vi "Testing.vi"() -> ()   [LabVIEW 2021]
uses:
  typeDefs/Esophogeal_Software_States.ctl
  <vilib>/Utility/miscctls.llb/LVAllMonitorsDisplayTypeDef.ctl
  <vilib>/DAQmx/read.llb/DAQmx Read (Digital 1D Bool NChan 1Samp 1Line).vi
  <extravilib>/ChannelInstances/Tag-bool/Read With Abort.vi
  <extravilib>/ChannelInstances/High Speed Stream-str/_Read For Replicate.vi
  <extravilib>/ChannelInstances/High Speed Stream-a[.,.](u32)/_Read For Replicate.vi
  <extravilib>/ChannelInstances/Tag-bool/Write With Abort.vi
  <extravilib>/ChannelInstances/High Speed Stream-a[.,.](u8)/_Read For Replicate.vi
  <vilib>/DAQmx/create/channels.llb/DAQmx Create Channel (DI-Digital Input).vi
  <extravilib>/ChannelInstances/Tag-bool/Instantiate.vi
  <extravilib>/ChannelInstances/Tag-bool/EndpointRead.vi
  <extravilib>/ChannelInstances/High Speed Stream-str/Instantiate.vi
  <extravilib>/ChannelInstances/High Speed Stream-a[.,.](u32)/Instantiate.vi
  <extravilib>/ChannelInstances/High Speed Stream-str/)Channel.vi
  <extravilib>/ChannelInstances/High Speed Stream-str/Abort Signal/Init Signal.vi
  <extravilib>/ChannelInstances/High Speed Stream-a[.,.](u32)/)Channel.vi
  <extravilib>/ChannelInstances/High Speed Stream-a[.,.](u32)/Abort Signal/Init Signal.vi
  <vilib>/DAQmx/miscellaneous.llb/DAQmx Fill In Error Info.vi
  <extravilib>/ChannelInstances/Tag-bool/Endpoint.vi
  <extravilib>/ChannelInstances/High Speed Stream-a[.,.](u8)/Instantiate.vi
  <extravilib>/ChannelInstances/High Speed Stream-a[.,.](u8)/)Channel.vi
  <extravilib>/ChannelInstances/High Speed Stream-a[.,.](u8)/Abort Signal/Init Signal.vi
  <vilib>/vision/driver/NI_Vision_Acquisition_Software.lvlib
  <resource>/objmgr/imaqdx.rc
  <extravilib>/ChannelInstances/High Speed Stream-a[.,.](u8).lvlib
  <extravilib>/ChannelInstances/High Speed Stream-str.lvlib
  <vilib>/vision/NI_Vision_Development_Module.lvlib
  <extravilib>/ChannelInstances/High Speed Stream-a[.,.](u32).lvlib
  <extravilib>/ChannelInstances/Tag-bool.lvlib
panel:
  out "Pause Status":bool
  in  "Tab Control":enum32{"Main Page", "Image Session Info"}(tab)
  in  "MTN Threshold:":enum16{"15.9", "24.0"}(ring)
  out "Endoscope Feed":T1(plugin-control)
  in  "Calibrate":bool
  out "Image Analysis Meter":dbl(slide) scale=0.0..100.0
  out "Saved Imaged Number":i32=1 caption="Number of Images Saved"
  out "Image Save Notification":string
  in  "Auto Gain":bool=TRUE
  in  "Auto Exposure":bool=TRUE
  in  "Save Button":bool
  out "Recording":bool
  in  "Play Button":bool
  in  "Pause Button":bool
  in  "Close Program":bool
  in  "HRME Gain":dbl(slide)=18.0 scale=0.0..30.0
  in  "HRME Exposure":dbl(slide)=7000.0 scale=100.0..80000.0
  out "HRME Image":T1(plugin-control)
  out "Software States":T2
  out "HRME Path":path
  out "HRME Scores":path
  out "Representative Images":path
  out "error out":errorcluster
  out "Patient Folder":path
  in  "Command File Location":path=path "C:/Users/EsophaHRME_Dell2/Documents/GitHub/Esophageal_HRME_Software/EsophagealDeployment/Multi_Task_Network/CommandFiles/LabVIEW/cmds.json"
  out "Display:All Monitors":T3
  out "Width":i16
  out "Height":i16=960
  out "WideField Path":path
  in  "Python Module Path":path=path "C:/Users/EsophaHRME_Dell2/Documents/GitHub/Esophageal_HRME_Software/EsophagealDeployment/Multi_Task_Network/mainv6.py"
  out "Log File Out":refnum<file>
  out "Timestamp":string
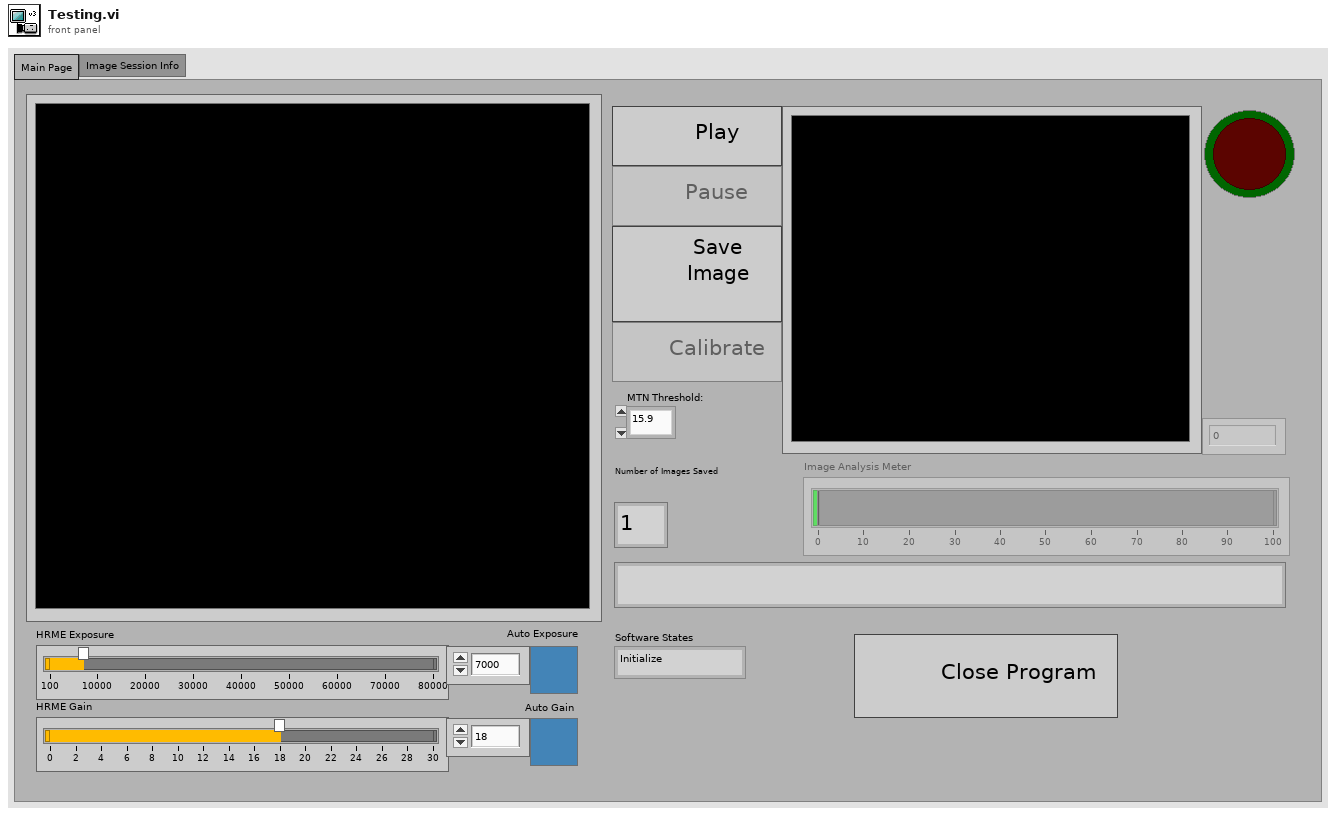
[diagram p1: front panel]
types:
  T1 = typedef "IMAQ Image.ctl" = refnum<image>
  T2 = typedef "Esophogeal_Software_States.ctl" = enum16{"Initialize", "Image Prep Screen", "Imaging", "Image Pause Screen", "Endo Only Saving", "Exit"}
  T3 = typedef "LVAllMonitorsDisplayTypeDef.ctl" = cluster{"Bounds":cluster{"Left":i16, "Top":i16, "Right":i16, "Bottom":i16}, "Depth":i16}[]
  T4 = enum8{"Enabled", "Disabled", "Disabled and Grayed Out"}
  T5 = enum16{"open", "replace", "create", "open or create", "replace or create", "replace or create with confirmation"}
  T6 = cluster{"Source":string, "Destination":string, "CMD":string, "Time":string}
  T7 = cluster{"Left":i32, "Top":i32, "Right":i32, "Bottom":i32}
  T8 = typedef "IMAQdx.ctl" = refnum<k21>
  T9 = cluster{"Bounds":cluster{"Left":i16, "Top":i16, "Right":i16, "Bottom":i16}, "Depth":i16}
  T10 = cluster{"Left":i16, "Top":i16, "Right":i16, "Bottom":i16}
  T11 = typedef "Image Type" = u32
  T12 = typedef "Tag-bool.lvlib/))Channel.ctl" = refnum<queue>
  T13 = typedef "ROI Descriptor" = cluster{"Global Rectangle":i32[], "Contours":cluster{"ID":enum32{"External", "Internal"}, "Type":u32, "Coordinates":i32[]}[]}
  T14 = typedef "High Speed Stream-a[.,.](u32).lvlib/)Channel.ctl" = refnum<queue>
  T15 = typedef "High Speed Stream-str.lvlib/)Channel.ctl" = refnum<queue>
  T16 = typedef "High Speed Stream-a[.,.](u8).lvlib/)Channel.ctl" = refnum<queue>
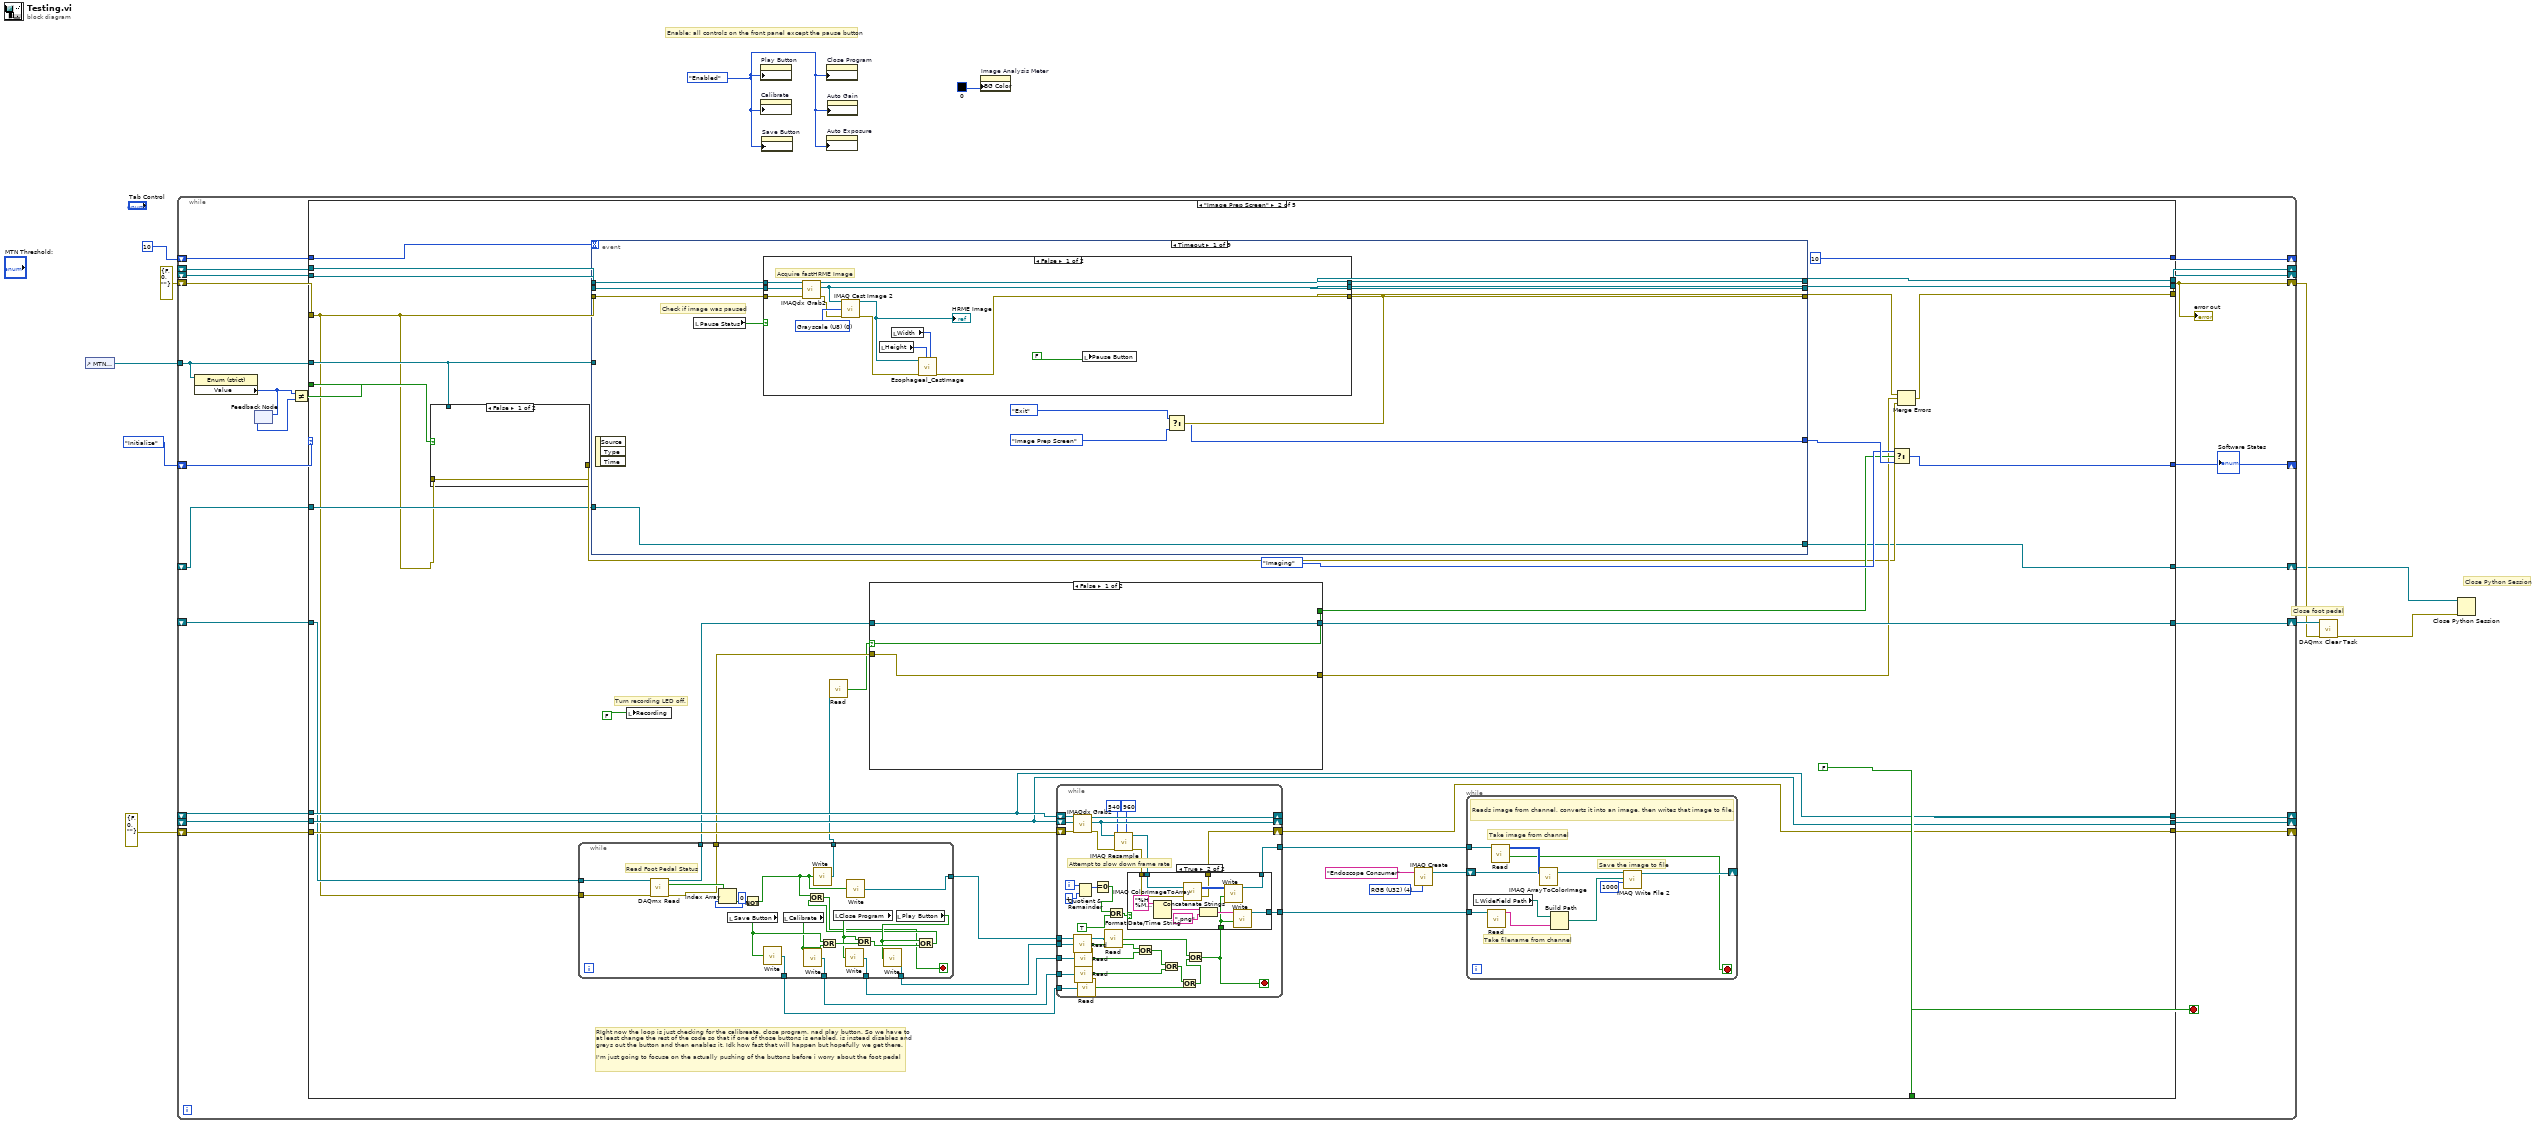
[diagram p0: block diagram]
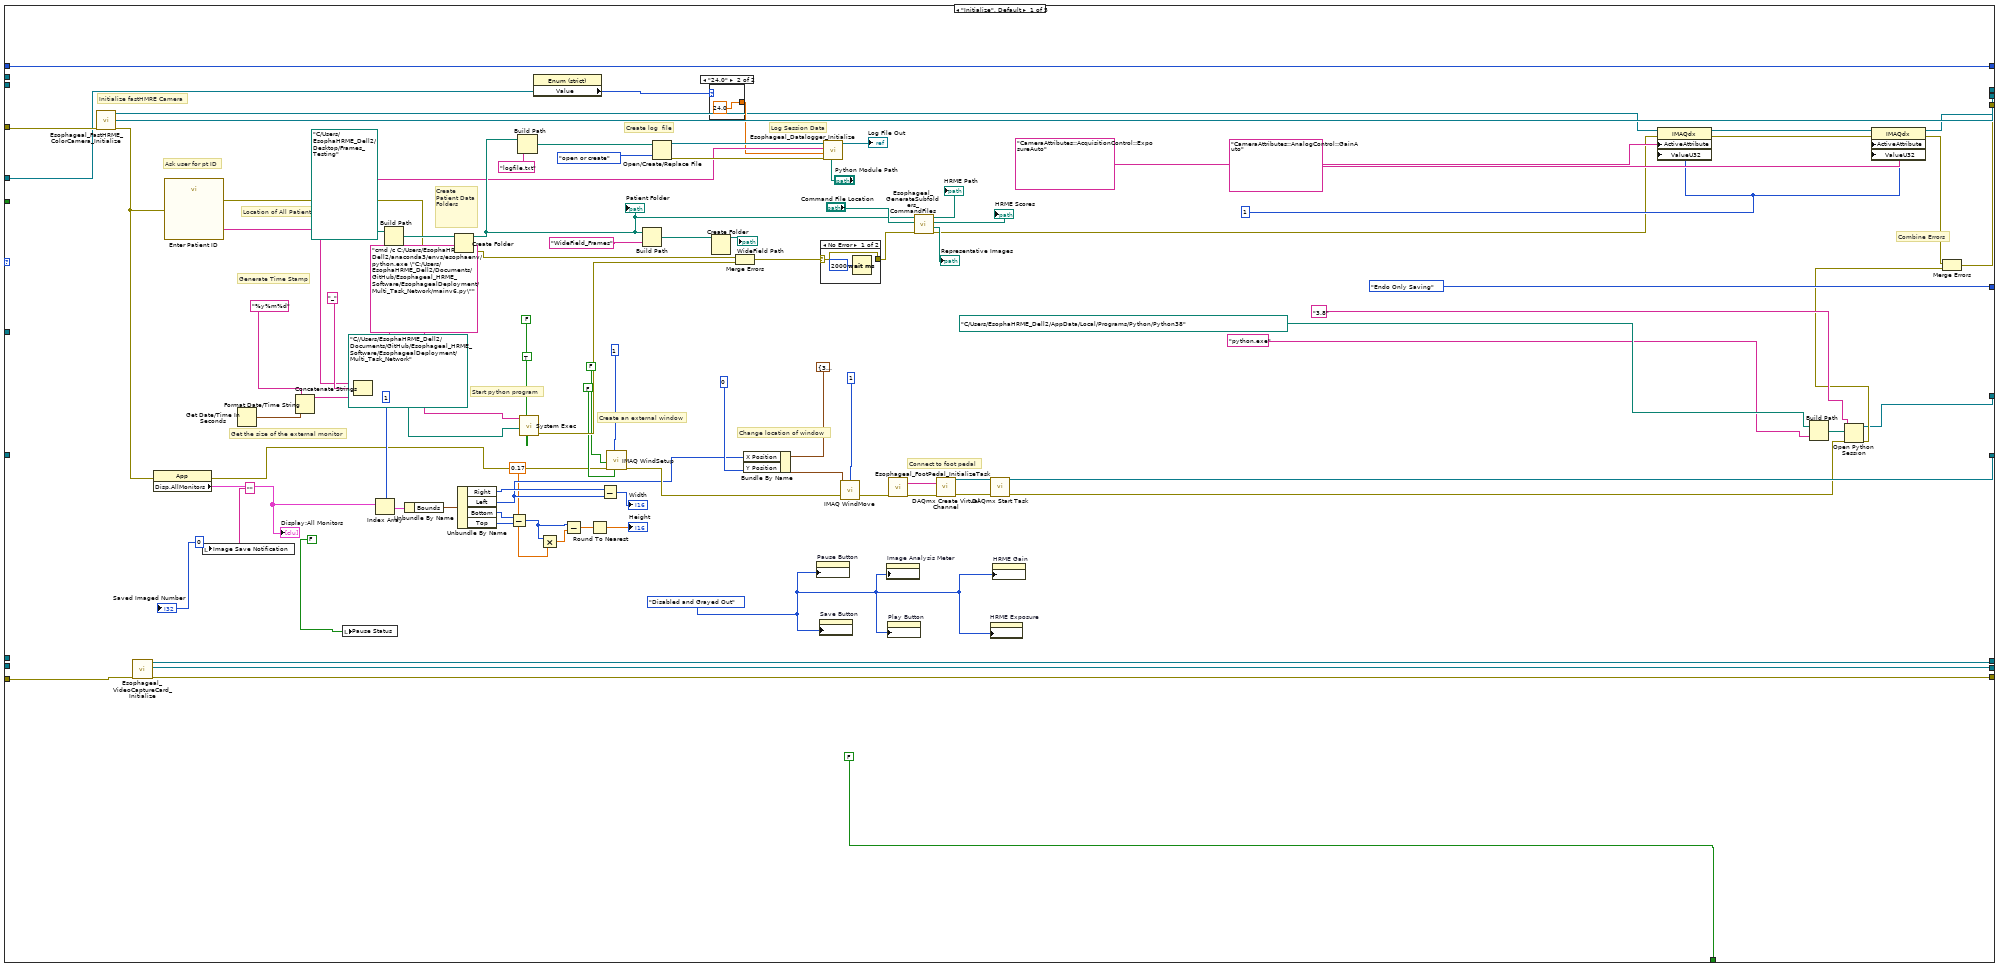
[diagram p2: hidden frame]
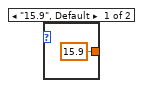
[diagram p3: hidden frame]
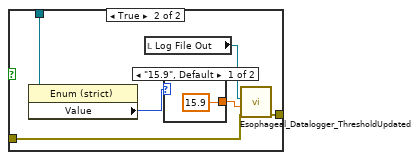
[diagram p6: hidden frame]
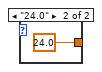
[diagram p7: hidden frame]
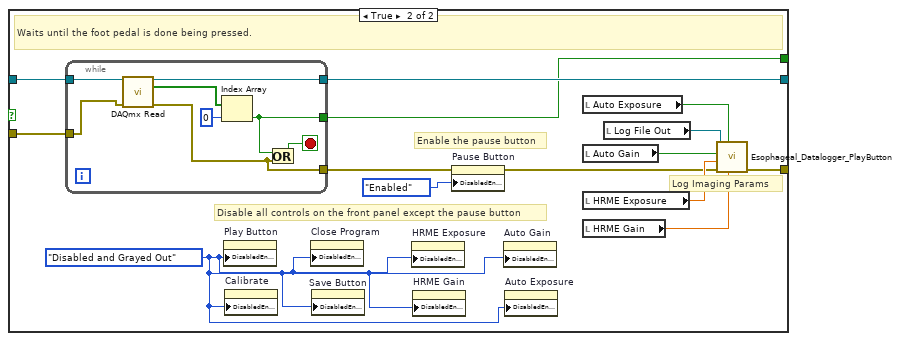
[diagram p8: hidden frame]
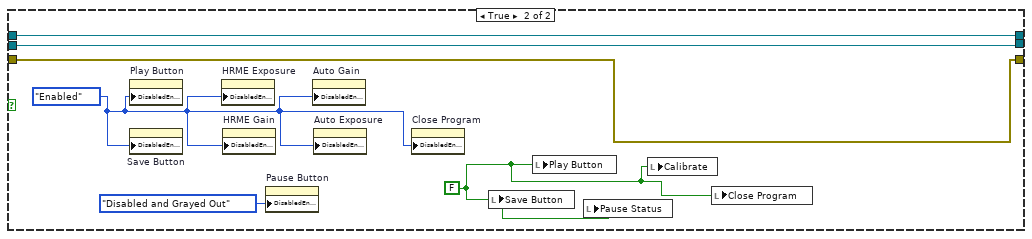
[diagram p9: hidden frame]
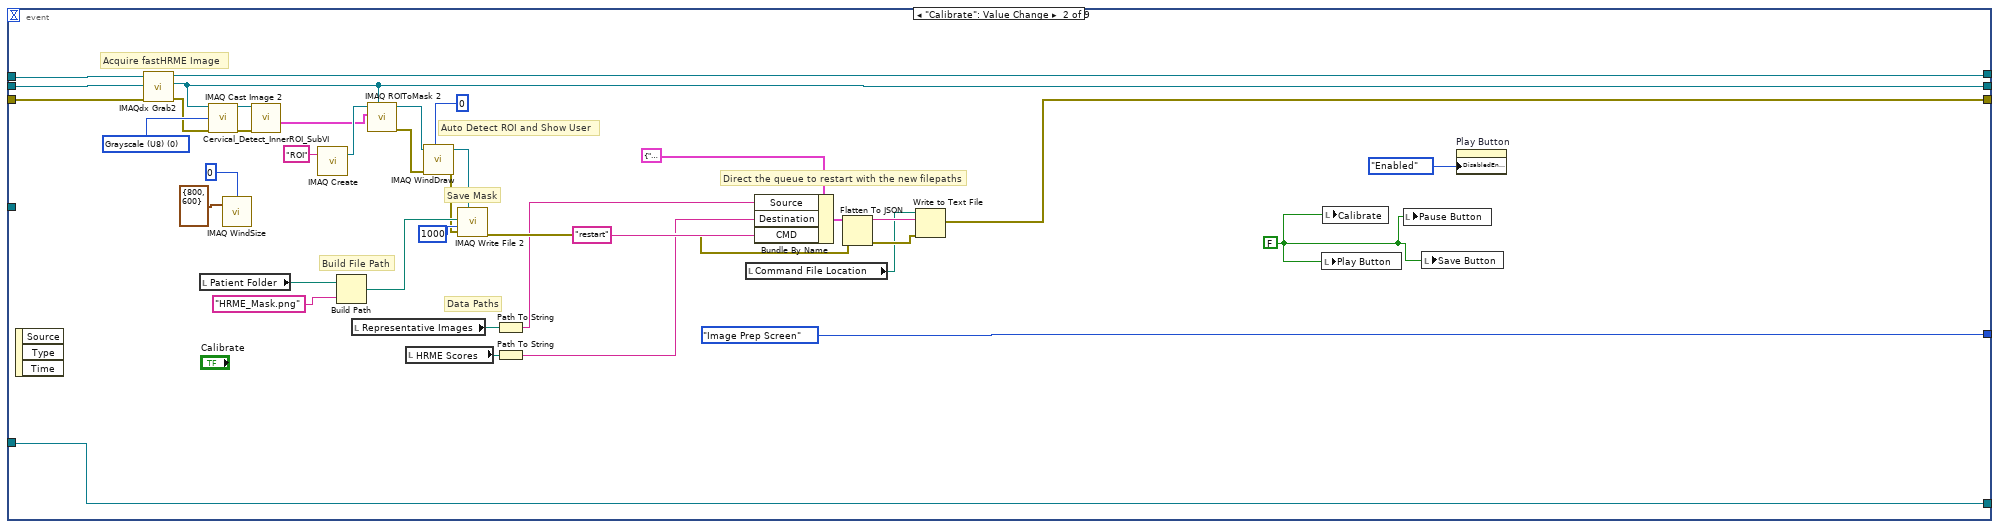
[diagram p10: hidden frame]
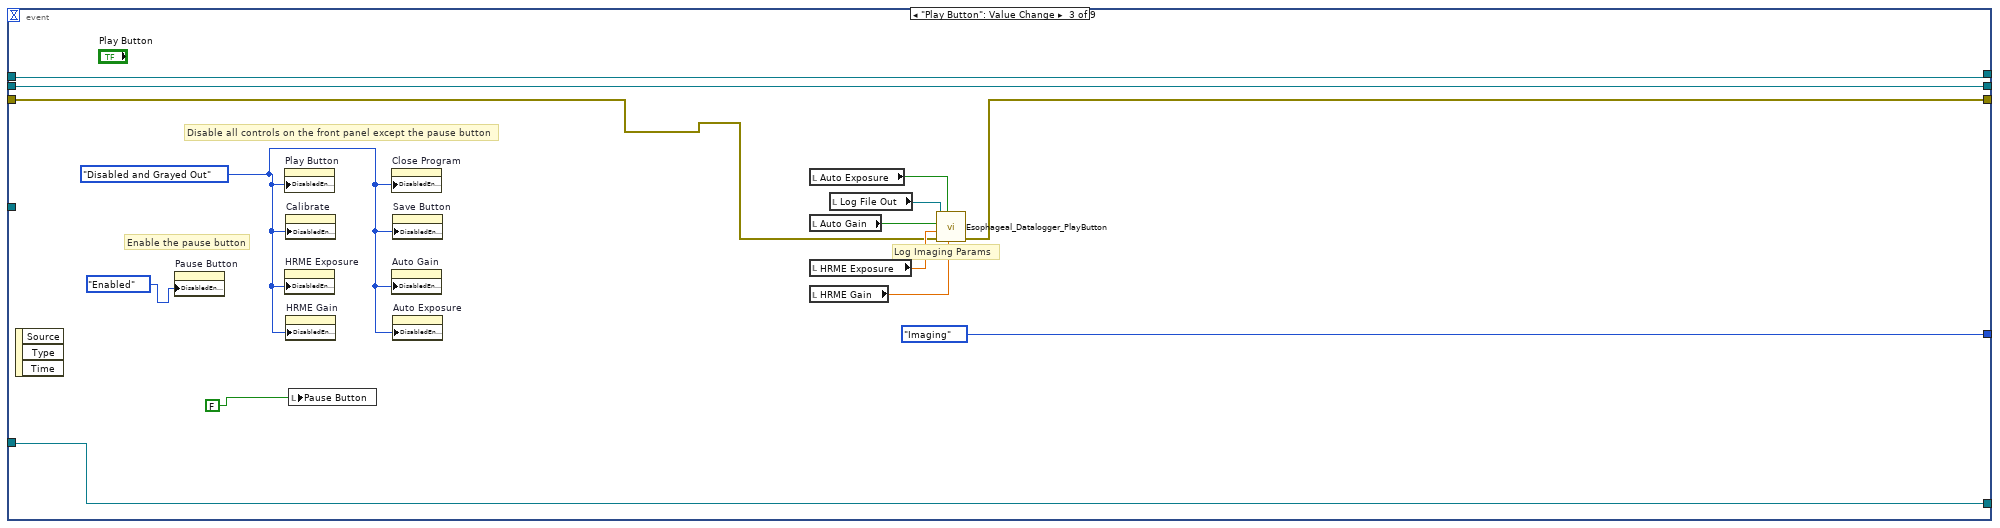
[diagram p11: hidden frame]
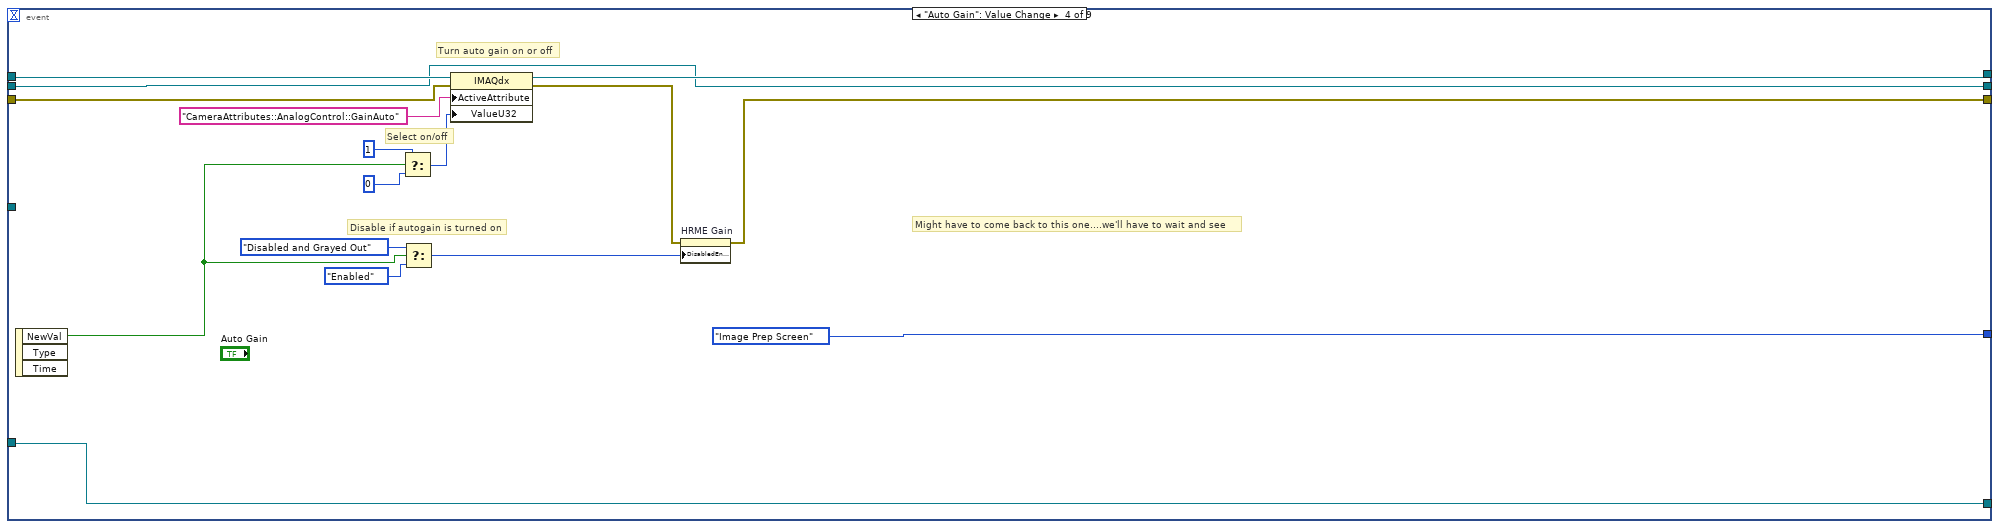
[diagram p12: hidden frame]
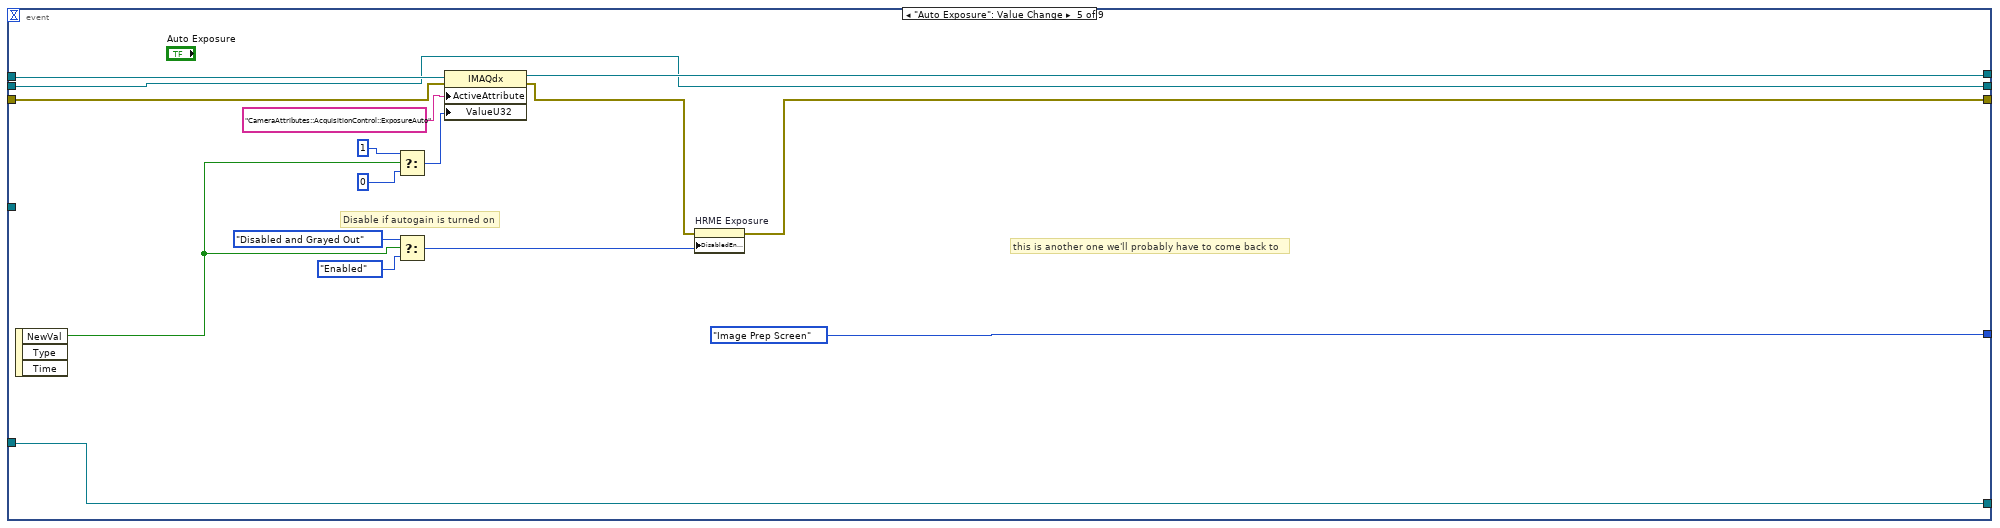
[diagram p13: hidden frame]
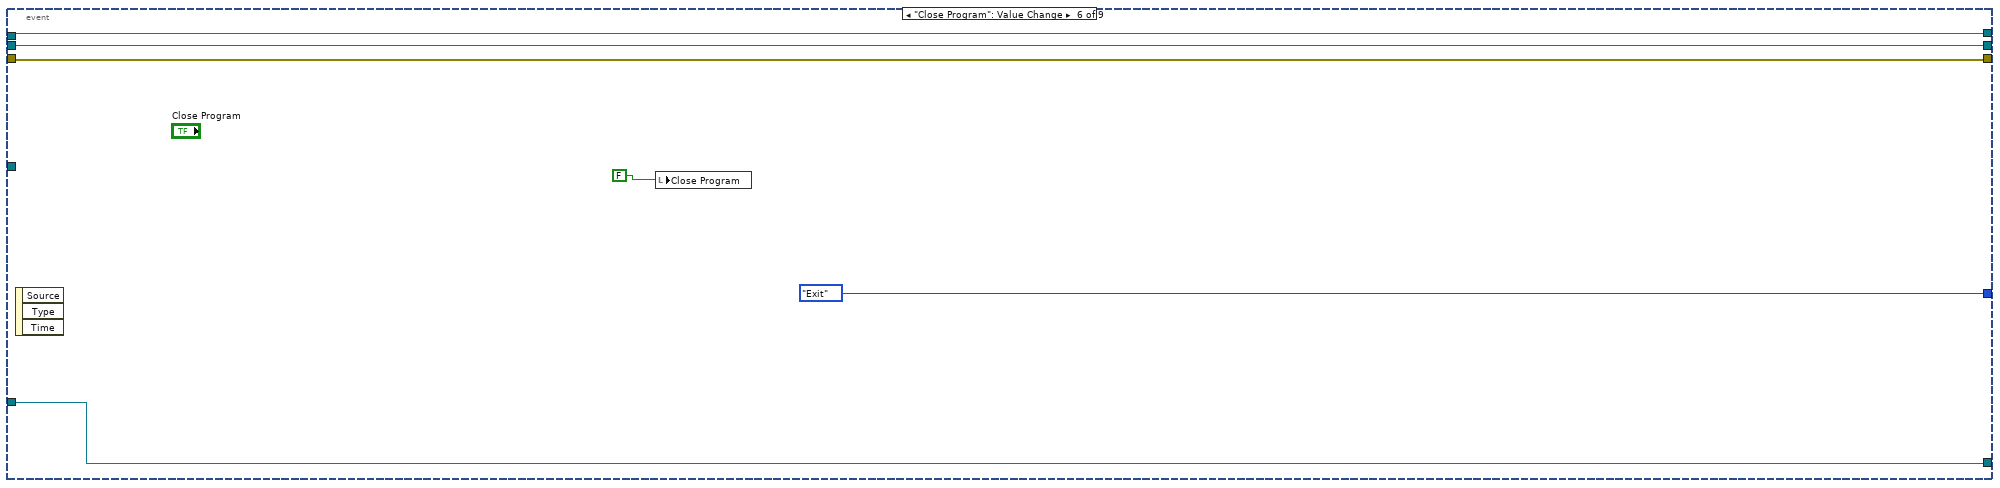
[diagram p14: hidden frame]
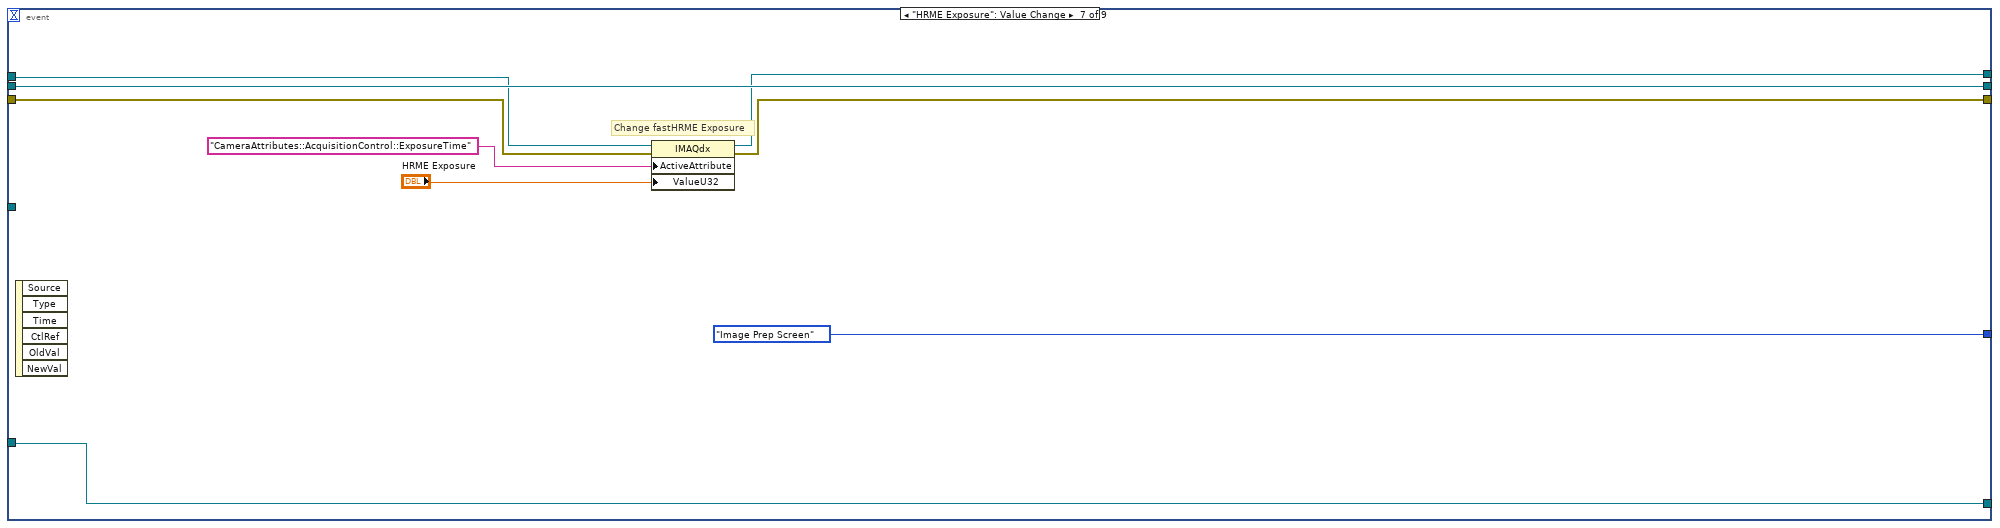
[diagram p15: hidden frame]
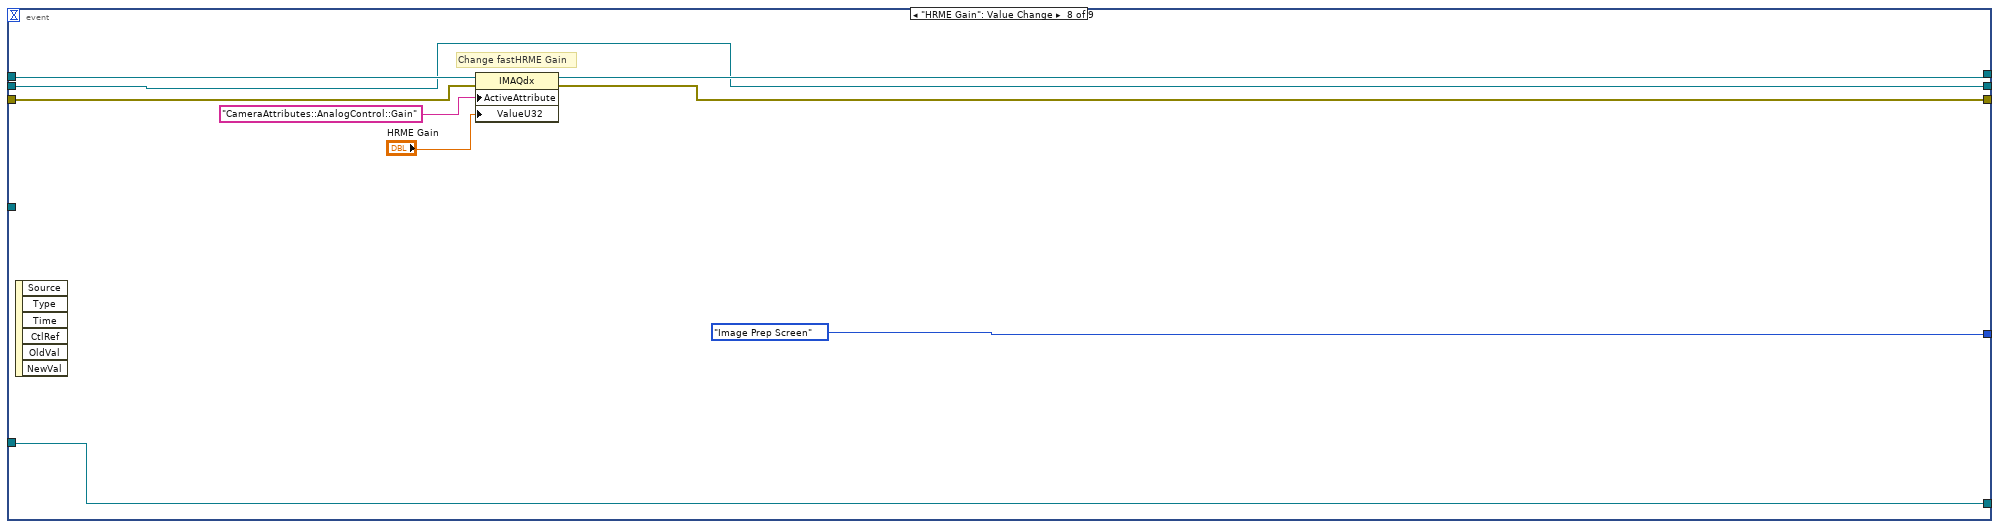
[diagram p16: hidden frame]
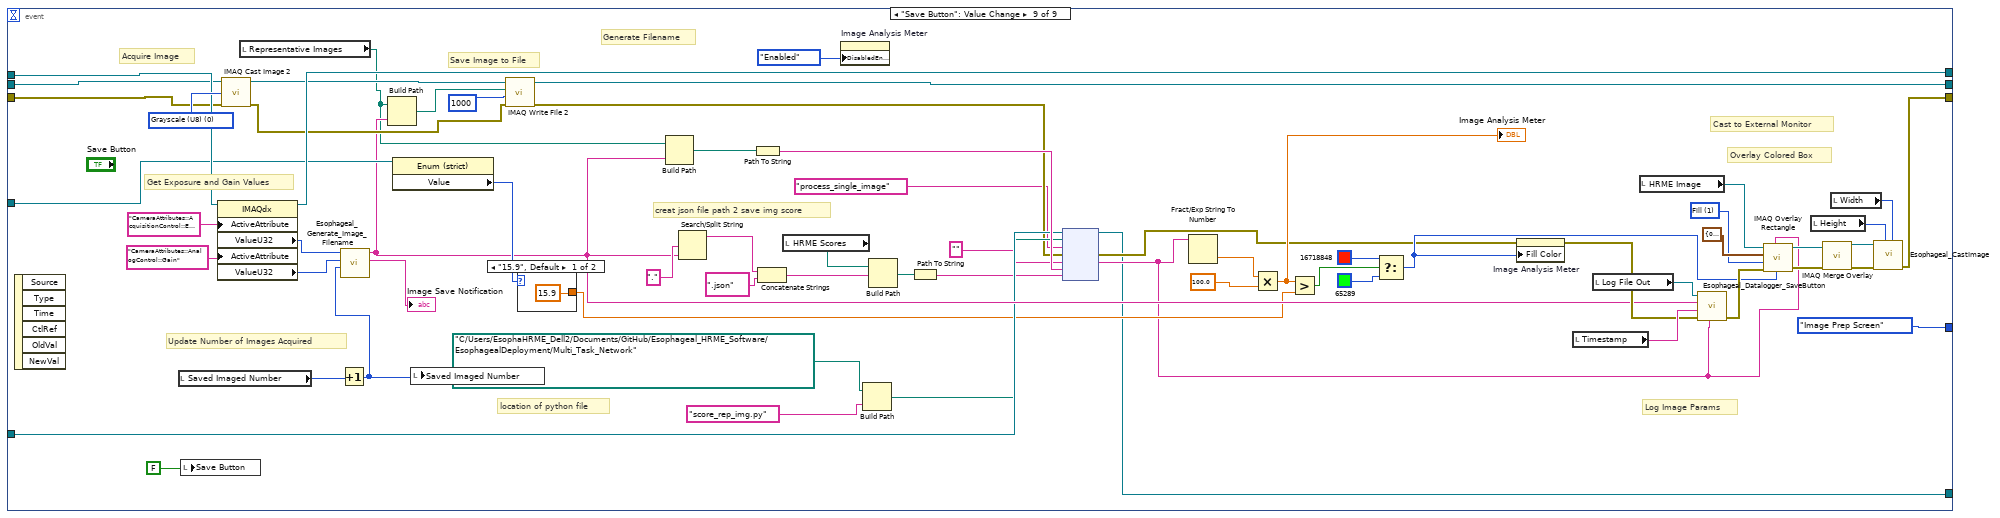
[diagram p17: hidden frame]
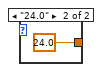
[diagram p18: hidden frame]
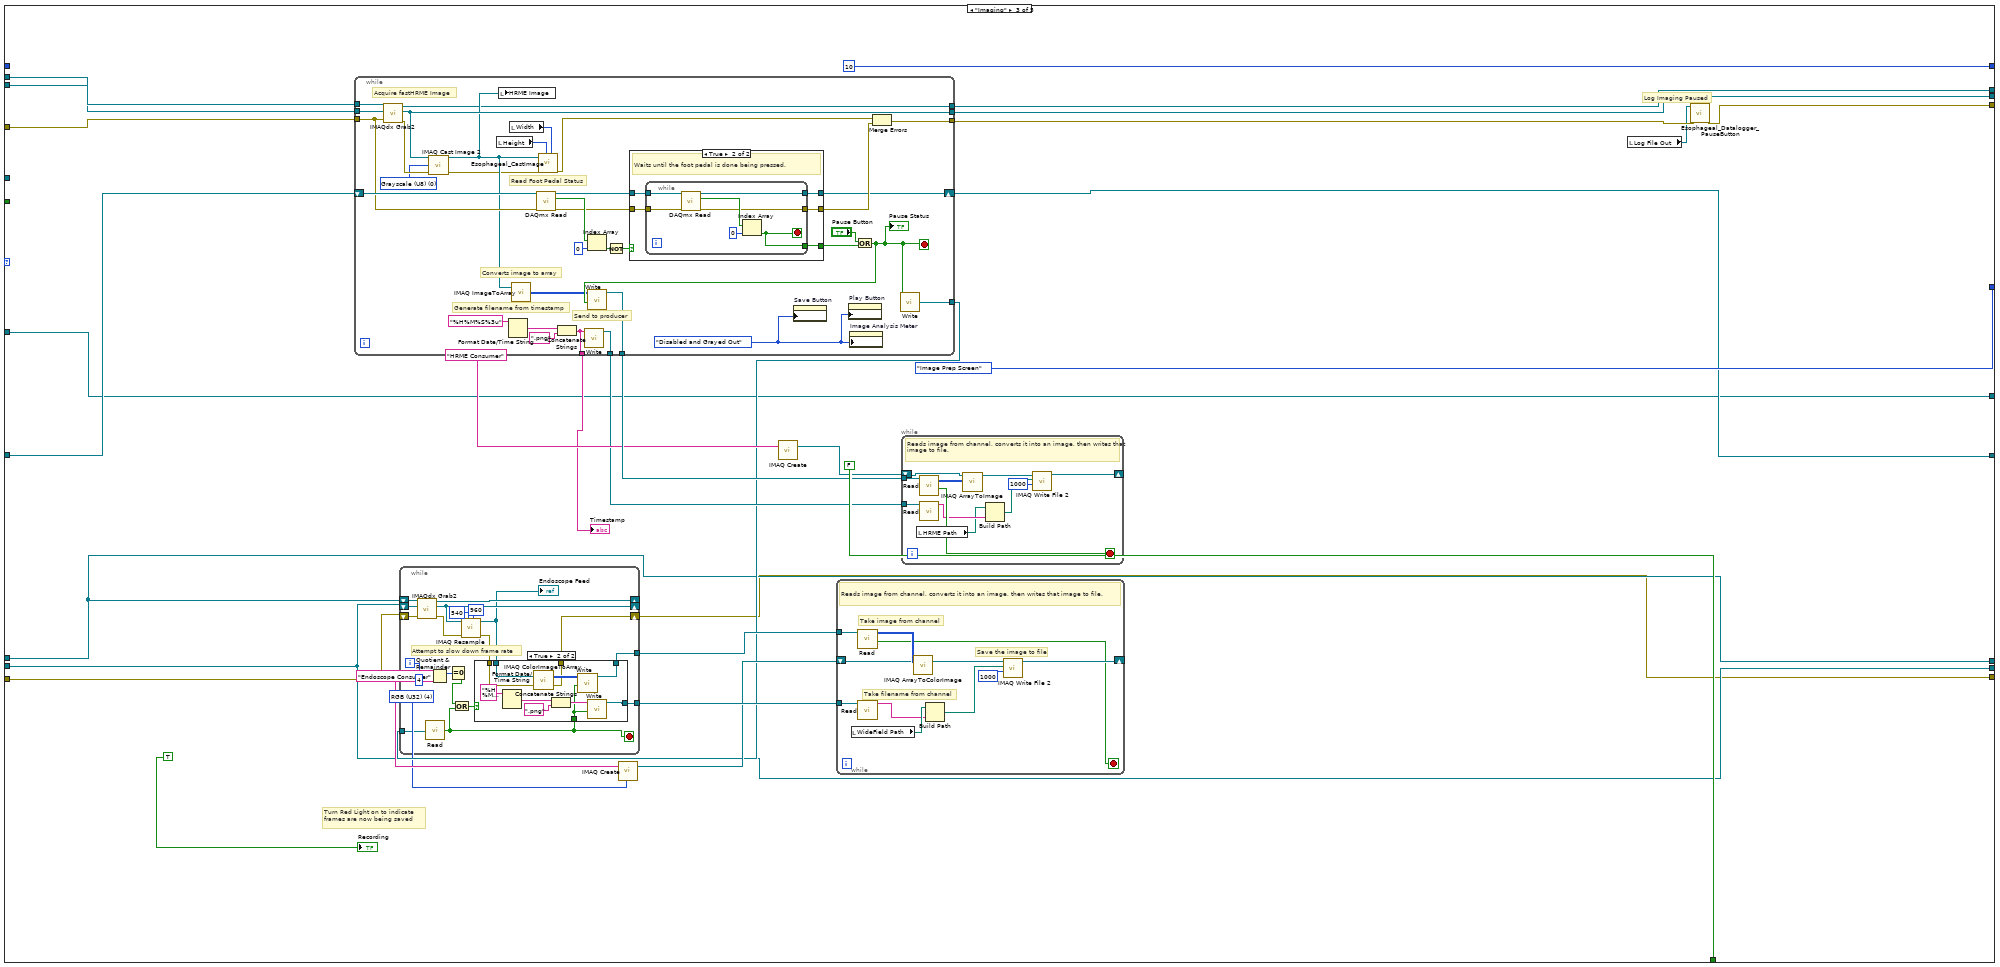
[diagram p19: hidden frame]
diagram:
  w3 = T4."Enabled" ("Disabled")
  # "Close Python Session"
  # "Enable; all controls on the front panel except the pause button"
  # "Close foot pedal"
  n1 = control-ref of="MTN Threshold:"() -> (w4:refnum<vi>)
  n2 = while {
    shift-right: [w35] -> _
    shift-left: _ -> [w32]
    shift-right: [w34] -> _
    shift-left: _ -> [w31]
    shift-right: [w33] -> _
    shift-left: Esophogeal_Software_States."Initialize" ("Anal HRME States") -> [w36]
    shift-right: [w25] -> w9
    shift-left: errorcluster {"status"=FALSE, "code"=0, "source"=""} ("error IO") -> [w24]
    shift-right: [w28] -> w10
    shift-left: _ -> [w29]
    shift-right: [w26] -> _
    shift-left: 10 -> [w27]
    shift-right: [w21] -> _
    shift-left: _ -> [w22]
    shift-right: [w20] -> _
    shift-left: _ -> [w23]
    shift-right: [w18] -> _
    shift-left: errorcluster {"status"=FALSE, "code"=0, "source"=""} ("error in (no error)") -> [w19]
    tunnel: w4 -> [w17]
    shift-right: [w13] -> w2
    shift-left: _ -> [w12]
    stop <- w30 stop-if-true
    n3 = property class="Enum (strict)"(reference=w17) -> ("Value"=w16:enum16{"15.9", "24.0"})  [unwired: 1 in, 2 out]
    n4 = feedback-in #1(w16) -> ()
    n5 = feedback #1() -> (w15:enum16{"15.9", "24.0"})  [unwired: 1 in]
    n6 = Not Equal?(x=w16, y=w15) -> (x != y?=w14:bool)
    n7 = case shown="\"Image Prep Screen\"" w36 {
      tunnel: [w46 w175 w521 w639 w742] -> w35
      tunnel: [w131 w174 w520 w638 w741] -> w34
      tunnel: [Esophogeal_Software_States."Endo Only Saving" ("Anal HRME States") w172 Esophogeal_Software_States."Image Prep Screen" ("Anal HRME States") Esophogeal_Software_States."Image Prep Screen" ("Anal HRME States") Esophogeal_Software_States."Exit" ("Anal HRME States")] -> w33
      tunnel: w24 -> [w129 w142 w505 w640 w731]
      tunnel: w32 -> [_ w177 w523 w642 w742]
      tunnel: w31 -> [_ w176 w522 w641 w741]
      tunnel: [FALSE FALSE FALSE FALSE TRUE] -> w30
      tunnel: [w114 w162 w503 w637 w729] -> w25
      tunnel: w29 -> [_ w143 w519 w634 w739]
      tunnel: [w125 w168 w516 w634 w739] -> w28
      tunnel: w27 -> [w124 w166 _ w653 w738]
      tunnel: [w124 10 10 w653 w738] -> w26
      tunnel: w19 -> [w65 w149 w500 w643 w725]
      tunnel: w23 -> [_ w146 w498 w645 w726]
      tunnel: w22 -> [_ w147 w499 w646 w727]
      tunnel: [w62 w146 w498 w645 w726] -> w20
      tunnel: [w63 w147 w499 w646 w727] -> w21
      tunnel: [w64 w148 w497 w632 w725] -> w18
      tunnel: w17 -> [w61 w159 _ _ _]
      tunnel: w14 -> [_ w160 _ _ _]
      tunnel: [w37 w157 w496 w633 w724] -> w13
      tunnel: w12 -> [_ w158 w496 w633 w724]
      frame "Initialize", Default {
        w50 = 1
        w44 = T4."Disabled and Grayed Out" ("Disabled")
        # "Log Session Data"
        # "Create log  file"
        # "Change location of window"
        # "Create an external window"
        # "Get the size of the external monitor"
        # "Start python program"
        # "Location of All Patient Data"
        # "Combine Errors"
        # "Create Patient Data Folders"
        # "Generate Time Stamp"
        # "Ask user for pt ID"
        # "Connect to foot pedal"
        # "Initialize fastHMRE Camera"
        n8 = call "Esophageal_FastHRME_ColorCamera_Initialize.vi"("error in (no error)"=w129) -> ("error out"=w91:errorcluster, "HRME Image Reference"=w131:T1, "OMS Camera Reference Out"=w47:T8)  [unwired: 8 in]
        n9 = call "Esophageal_VideoCaptureCard_Initialize.vi"("error in (no error)"=w65) -> ("error out"=w64:errorcluster, "Capture Card Image Out"=w62:T1, "Capture Card Camera Out"=w63:T8)  [unwired: 8 in]
        n10 = property class="App"(error in=w91) -> (error out=w80:errorcluster, "Disp.AllMonitors"=w98:T3)  [unwired: 1 in, 1 out]
        "Display:All Monitors" <- w98
        n11 = call "Enter Patient ID"("error in (no error)"=w91) -> ("Patient ID"=w66:string, "error out"=w115:errorcluster)  [unwired: 16 in, 1 out]
        n12 = local write "Image Save Notification"("" ("Image Save Notification")) -> ()
        n13 = Get Date/Time In Seconds() -> (seconds since 1Jan1904=w121:timestamp)
        n14 = Format Date/Time String(time format string (%c)="%y%m%d", seconds (now)=w121) -> (date/time string=w118:string)  [unwired: 1 in]
        n15 = local write "Pause Status"(FALSE ("Pause Status")) -> ()
        n16 = Concatenate Strings(w66, "_" ("string"), w118) -> (w117:string)
        n17 = Index Array(array=w98, index=1) -> (element=w96:T9)
        n18 = Build Path(base path=path "C:/Users/EsophaHRME_Dell2/Desktop/Frames_Testing", name or relative path=w117) -> (appended path=w116:path)
        n19 = Unbundle By Name(w96) -> ("Bounds"=w95:T10)
        n20 = Create Folder(path (use dialog)=w116, error in=w115) -> (created path=w68:path, error out=w78:errorcluster)  [unwired: 1 in, 1 out]
        "Patient Folder" <- w68
        n21 = Unbundle By Name(w95) -> ("Right"=w94:i16, "Left"=w79:i16, "Bottom"=w93:i16, "Top"=w92:i16)
        n22 = Subtract(x=w93, y=w92) -> (x-y=w57:i16)
        n23 = Build Path(base path=w68, name or relative path="logfile.txt") -> (appended path=w74:path)
        n24 = call <vilib>:"System Exec.vi"("run minimized? (F)"=TRUE, "wait until completion? (T)"=FALSE, "working directory"=path "C://Users/EsophaHRME_Dell2/Documents/GitHub/Esophageal_HRME_Software/EsophagealDeployment/Multi_Task_Network", "command line"="cmd /c C:/Users/EsophaHRME_Dell2/anaconda3/envs/esophaenv/python.exe \"C:/Users/EsophaHRME_Dell2/Documents/GitHub/Esophageal_HRME_Software/EsophagealDeployment/Multi_Task_Network/mainv6.py\"") -> ("error out"=w103:errorcluster)  [unwired: 4 in, 3 out]
        n25 = property class="Enum (strict)"(reference=w61) -> ("Value"=w60:enum16{"15.9", "24.0"})  [unwired: 1 in, 2 out]
        n26 = Multiply(x=w57, y=0.17) -> (x*y=w56:dbl)
        n27 = Subtract(x=w57, y=w56) -> (x-y=w55:dbl)
        n28 = Round To Nearest(number=w55) -> (nearest integer value=→"Height":dbl)
        n29 = Subtract(x=w94, y=w79) -> (x-y=→"Width":i16)
        n30 = call "IMAQ WindSetup"("Window is floating? (No)"=FALSE, "Window Number (0...15)"=1, "error in (no error)"=w80, "Window has title bar? (Yes)"=FALSE) -> ("error out"=w81:errorcluster)  [unwired: 7 in]
        n31 = Build Path(base path=w68, name or relative path="WideField_Frames") -> (appended path=w76:path)
        n32 = Open/Create/Replace File(file path (use dialog)=w74, operation (0:open)=T5."open or create") -> (refnum out=w72:refnum<file>, error out=w71:errorcluster)  [unwired: 4 in, 1 out]
        n33 = case shown="\"24.0\"" w60 {
          tunnel: [15.9 24.0] -> w59
          frame "15.9", Default {
          }
          frame "24.0" {
          }
        }
        n34 = Create Folder(path (use dialog)=w76) -> (created path=→"WideField Path":path)  [unwired: 2 in, 2 out]
        n35 = Merge Errors(w78, w103) -> (w104:errorcluster)
        n36 = Bundle By Name(cluster=cluster{"X Position":i32, "Y Position":i32} {"X Position"=3840, "Y Position"=0} ("Coordinates (screen)"), "X Position"=w79, "Y Position"=0) -> (w86:cluster{"X Position":i32, "Y Position":i32})
        n37 = property on="Pause Button" class="Bool (strict)"("DisabledEnum"=w44) -> ()  [unwired: 2 in, 2 out]
        n38 = property on="Save Button" class="Bool (strict)"("DisabledEnum"=w44) -> ()  [unwired: 2 in, 2 out]
        n39 = case shown="No Error" w104 {
          selector: w104 -> [w134 w136]
          tunnel: [w134 w136] -> w108
          frame No Error {
            n40 = Wait (ms)(milliseconds to wait=u32 2000) -> ()  [unwired: 1 out]
          }
          frame Error {
          }
        }
        n41 = call "Esophageal_Datalogger_Initialize.vi"("Python Module Path"="Python Module Path", "error in (no error)"=w71, "MTN Threshold"=w59, "Patient ID"=w66, "Log File In"=w72) -> ("Log File Out"=→"Log File Out":refnum<file>)  [unwired: 5 in, 1 out]
        n42 = call "IMAQ WindMove"("Window Number (0...15)"=1, "Coordinates (screen)"=w86, "error in (no error)"=w81) -> ("error out"=w82:errorcluster)  [unwired: 2 in, 1 out]
        n43 = property on="Image Analysis Meter" class="Slide (strict)"("DisabledEnum"=w44) -> ()  [unwired: 2 in, 2 out]
        n44 = property on="Play Button" class="Bool (strict)"("DisabledEnum"=w44) -> ()  [unwired: 2 in, 2 out]
        n45 = call "Esophageal_FootPedal_InitializeTask.vi"("error in (no error)"=w82) -> ("error out"=w101:errorcluster, "Task Command"=w100:string)  [unwired: 9 in]
        n46 = call "Esophageal_GenerateSubfolders_CommandFiles.vi"("error in"=w108, "Command File Location"="Command File Location", "Patient Data Folder"=w68) -> ("error out"=w48:errorcluster, "Rep Image Path"=→"Representative Images":path, "HRME Scores"=→"HRME Scores":path, "HRME Path"=→"HRME Path":path)  [unwired: 5 in]
        n47 = call-poly <vilib>:"DAQmx Create Virtual Channel.vi"("lines"=w100, "error in"=w101) -> ("task out"=w126:refnum<k21>, "error out"=w127:errorcluster)  [unwired: 12 in]
        n48 = property on="HRME Exposure" class="Slide (strict)"("DisabledEnum"=w44) -> ()  [unwired: 2 in, 2 out]
        n49 = call <vilib>:"DAQmx Start Task.vi"("task/channels in"=w126, "error in"=w127) -> ("task out"=w125:refnum<k21>, "error out"=w39:errorcluster)  [unwired: 12 in]
        n50 = property on="HRME Gain" class="Slide (strict)"("DisabledEnum"=w44) -> ()  [unwired: 2 in, 2 out]
        n51 = property class="IMAQdx"(reference=w47, error in=w48, "ActiveAttribute"="CameraAttributes::AcquisitionControl::ExposureAuto", "ValueU32"=w50) -> (reference out=w49:T8, error out=w51:errorcluster)
        n52 = Build Path(base path=path "C:/Users/EsophaHRME_Dell2/AppData/Local/Programs/Python/Python38", name or relative path="python.exe") -> (appended path=w42:path)
        n53 = Open Python Session(python version="3.8", python path=w42, 3:w39) -> (session out=w37:refnum<k35>, error out=w38:errorcluster)
        n54 = property class="IMAQdx"(reference=w49, error in=w51, "ActiveAttribute"="CameraAttributes::AnalogControl::GainAuto", "ValueU32"=w50) -> (reference out=w46:T8, error out=w45:errorcluster)
        n55 = Merge Errors(w45, w38) -> (w114:errorcluster)
        "Saved Imaged Number" <- 0
      }
      frame "Image Prep Screen" {
        w152 = T11 4 items=["Grayscale (U8)", "Grayscale (I16)", "Grayscale (SGL)", "Complex (CSG)", "RGB (U32)", "HSL (U32)", "RGB (U64)", "Grayscale (U16)"] ("Image Type")
        # "RIght now the loop is just checking for the calibreate, close program, nad play button. So we have to \nat least change the rest of the code so that if one of those buttons is enabled, is instead disables and \ngreys out the button and then enables it. Idk how fast that will happen but hopefully we get there. \n\nI'm just going to focuse on the actually pushing of the buttons before i worry about the foot pedal"
        # "Turn recording LED off."
        n56 = case shown="False" w160 {
          tunnel: w142 -> [w256 w260]
          tunnel: [w256 w259] -> w161
          tunnel: w159 -> [_ w257]
          frame False {
          }
          frame True {
            n57 = property class="Enum (strict)"(reference=w257) -> ("Value"=w262:enum16{"15.9", "24.0"})  [unwired: 1 in, 2 out]
            n58 = local read "Log File Out"() -> (w258:refnum<file>)
            n59 = case shown="\"15.9\", Default" w262 {
              tunnel: [15.9 24.0] -> w261
              frame "15.9", Default {
              }
              frame "24.0" {
              }
            }
            n60 = call "Esophageal_Datalogger_ThresholdUpdated.vi"("error in"=w260, "MTN Threshold"=w261, "Log File In"=w258) -> ("error out"=w259:errorcluster)  [unwired: 7 in, 1 out]
          }
        }
        n61 = while {
          tunnel: [w199] -> w151
          tunnel: [w198] -> w150
          tunnel: [w197] -> w145
          tunnel: [w196] -> w144
          tunnel: w143 -> [w187]
          tunnel: w142 -> [w186]
          tunnel: [w184] -> w141
          tunnel: [w183] -> w140
          tunnel: [w180] -> w138
          tunnel: [w178] -> w139
          stop <- w181 stop-if-true
          # "Read Foot Pedal Status"
          n62 = call-poly <vilib>:"DAQmx Read.vi"("task/channels in"=w187, "error in"=w186) -> ("task out"=w184:refnum<k21>, "data"=w188:bool[], "error out"=w183:errorcluster)  [unwired: 11 in]
          n63 = Index Array(array=w188, index=0) -> (element=w189:bool)
          n64 = local read "Save Button"() -> (w195:bool)
          n65 = Not(x=w189) -> (.not. x?=w179:bool)
          n66 = call <extravilib>:"Write.vi"("element"=w195) -> ("channel"=w196:T12)  [unwired: 1 out]
          n67 = local read "Calibrate"() -> (w194:bool)
          n68 = call <extravilib>:"Write.vi"("element"=w194) -> ("channel"=w197:T12)  [unwired: 1 out]
          n69 = call <extravilib>:"Write.vi"("element"=w179) -> ("channel"=w180:T12)  [unwired: 1 out]
          n70 = Or(x=w195, y=w194) -> (x .or. y?=w193:bool)
          n71 = local read "Close Program"() -> (w192:bool)
          n72 = call <extravilib>:"Write.vi"("element"=w192) -> ("channel"=w199:T12)  [unwired: 1 out]
          n73 = call <extravilib>:"Write.vi"("element"=w179) -> ("channel"=w178:T12)  [unwired: 1 out]
          n74 = Or(x=w192, y=w193) -> (x .or. y?=w191:bool)
          n75 = local read "Play Button"() -> (w190:bool)
          n76 = call <extravilib>:"Write.vi"("element"=w190) -> ("channel"=w198:T12)  [unwired: 1 out]
          n77 = Or(x=w190, y=w191) -> (x .or. y?=w182:bool)
          n78 = Or(x=w179, y=w182) -> (x .or. y?=w181:bool)
        }
        n79 = event shown="[0] Timeout" {
          selector: _ -> [_ _ _ _ _ _ _ _ _]
          dyn-events: _ -> [_ _ _ _ _ _ _ _ _]
          timeout: w166 -> [_ _ _ _ _ _ _ _ _]
          tunnel: w177 -> [w300 w357 w371 w388 w401 w409 w417 w426 w478]
          tunnel: w176 -> [w298 w356 w370 w385 w398 w408 w418 w422 w477]
          tunnel: [w292 Esophogeal_Software_States."Image Prep Screen" ("Anal HRME States") Esophogeal_Software_States."Imaging" ("Anal HRME States") Esophogeal_Software_States."Image Prep Screen" ("Anal HRME States") Esophogeal_Software_States."Image Prep Screen" ("Anal HRME States") Esophogeal_Software_States."Exit" ("Anal HRME States") Esophogeal_Software_States."Image Prep Screen" ("Anal HRME States") Esophogeal_Software_States."Image Prep Screen" ("Anal HRME States") Esophogeal_Software_States."Image Prep Screen" ("Anal HRME States")] -> w171
          tunnel: [w299 w355 w371 w387 w400 w409 w416 w425 w488] -> w175
          tunnel: [w297 w335 w370 w385 w398 w408 w418 w422 w491] -> w174
          tunnel: w142 -> [w296 w323 w361 w386 w399 w407 w413 w423 w476]
          tunnel: [w293 w322 w364 w376 w394 w407 w412 w424 w473] -> w163
          tunnel: w159 -> [_ _ _ _ _ _ _ _ w460]
          tunnel: w158 -> [w290 w324 w363 w373 w389 w406 w411 w420 w446]
          tunnel: [w290 w324 w363 w373 w389 w406 w411 w420 w430] -> w157
          event Timeout {
            # "Check if image was paused"
            n80 = event-data() -> ()  [unwired: 1 in, 3 out]
            n81 = local read "Pause Status"() -> (w295:bool)
            n82 = case shown="False" w295 {
              tunnel: w300 -> [w313 w319]
              tunnel: [w312 w319] -> w299
              tunnel: w298 -> [w311 w318]
              tunnel: [w309 w318] -> w297
              tunnel: w296 -> [w310 w316]
              tunnel: [w304 w316] -> w293
              frame False {
                w308 = T11 0 items=["Grayscale (U8)", "Grayscale (I16)", "Grayscale (SGL)", "Complex (CSG)", "RGB (U32)", "HSL (U32)", "RGB (U64)", "Grayscale (U16)"] ("Image Type")
                # "Acquire fastHRME Image"
                n83 = call <vilib>:"IMAQdx Grab2.vi"("error in"=w310, "Image In"=w311, "Session In"=w313) -> ("error out"=w306:errorcluster, "Image Out"=w309:T1, "Session Out"=w312:T8)  [unwired: 5 in, 1 out]
                n84 = call "IMAQ Cast Image 2"("Image Src"=w309, "Image Type"=w308, "error in (no error)"=w306) -> ("Image Dst Out"=w307:T1, "error out"=w305:errorcluster)  [unwired: 11 in]
                "HRME Image" <- w307
                n85 = local read "Height"() -> (w303:i16)
                n86 = local read "Width"() -> (w302:i16)
                n87 = call "Esophageal_CastImage.vi"("X Resolution"=w302, "Y Resolution"=w303, "error in (no error)"=w305, "Image In"=w307) -> ("error out"=w304:errorcluster)  [unwired: 7 in]
                n88 = local write "Pause Button"(FALSE) -> ()
              }
              frame True {
                w314 = FALSE
                w315 = T4."Enabled" ("Disabled")
                n89 = property on="Play Button" class="Bool (strict)"("DisabledEnum"=w315) -> ()  [unwired: 2 in, 2 out]
                n90 = property on="Save Button" class="Bool (strict)"("DisabledEnum"=w315) -> ()  [unwired: 2 in, 2 out]
                n91 = property on="HRME Exposure" class="Slide (strict)"("DisabledEnum"=w315) -> ()  [unwired: 2 in, 2 out]
                n92 = property on="HRME Gain" class="Slide (strict)"("DisabledEnum"=w315) -> ()  [unwired: 2 in, 2 out]
                n93 = property on="Pause Button" class="Bool (strict)"("DisabledEnum"=T4."Disabled and Grayed Out" ("Disabled")) -> ()  [unwired: 2 in, 2 out]
                n94 = property on="Auto Gain" class="Bool (strict)"("DisabledEnum"=w315) -> ()  [unwired: 2 in, 2 out]
                n95 = property on="Auto Exposure" class="Bool (strict)"("DisabledEnum"=w315) -> ()  [unwired: 2 in, 2 out]
                n96 = property on="Close Program" class="Bool (strict)"("DisabledEnum"=w315) -> ()  [unwired: 2 in, 2 out]
                n97 = local write "Save Button"(w314) -> ()
                n98 = local write "Play Button"(w314) -> ()
                n99 = local write "Pause Status"(w314) -> ()
                n100 = local write "Calibrate"(w314) -> ()
                n101 = local write "Close Program"(w314) -> ()
              }
            }
            n102 = Select(t=Esophogeal_Software_States."Exit" ("Anal HRME States"), s=w293, f=Esophogeal_Software_States."Image Prep Screen" ("Anal HRME States")) -> (s? t:f=w292:T2)
          }
          event "Calibrate": Value Change {
            w320 = FALSE
            w358 = T11 0 items=["Grayscale (U8)", "Grayscale (I16)", "Grayscale (SGL)", "Complex (CSG)", "RGB (U32)", "HSL (U32)", "RGB (U64)", "Grayscale (U16)"] ("Image Type")
            # "Auto Detect ROI and Show User"
            # "Data Paths"
            # "Direct the queue to restart with the new filepaths"
            # "Build File Path"
            # "Save Mask"
            # "Acquire fastHRME Image"
            n103 = event-data() -> ()  [unwired: 1 in, 3 out]
            n104 = call <vilib>:"IMAQdx Grab2.vi"("error in"=w323, "Image In"=w356, "Session In"=w357) -> ("error out"=w347:errorcluster, "Image Out"=w335:T1, "Session Out"=w355:T8)  [unwired: 5 in, 1 out]
            n105 = local read "Patient Folder"() -> (w353:path)
            n106 = call "IMAQ Cast Image 2"("Image Src"=w335, "Image Type"=w358, "error in (no error)"=w347) -> ("Image Dst Out"=w326:T1, "error out"=w327:errorcluster)  [unwired: 11 in]
            n107 = call "IMAQ WindSize"("Width & Height"=cluster{"Width":i32, "Height":i32} {"Width"=800, "Height"=600}, "Window Number"=0) -> ()  [unwired: 4 in, 3 out]
            n108 = call "Cervical_Detect_InnerROI_SubVI.vi"("error in"=w327, "Raw Image"=w326) -> ("ROI Descriptor"=w325:T13)  [unwired: 6 in, 3 out]
            n109 = call "IMAQ Create"("Image Name"="ROI") -> ("New Image"=w348:T1)  [unwired: 4 in, 1 out]
            n110 = Build Path(base path=w353, name or relative path="HRME_Mask.png") -> (appended path=w351:path)
            n111 = local read "Representative Images"() -> (w339:path)
            n112 = call "IMAQ ROIToMask 2"("Image Model"=w335, "ROI Descriptor"=w325, "Image"=w348) -> ("error out"=w330:errorcluster, "Image Out"=w331:T1)  [unwired: 6 in, 1 out]
            n113 = local read "HRME Scores"() -> (w338:path)
            n114 = call "IMAQ WindDraw"("Window Number (0...15)"=0, "error in (no error)"=w330, "Image"=w331) -> ("error out"=w328:errorcluster, "Image Out (duplicate)"=w329:T1)  [unwired: 7 in]
            n115 = call-poly "IMAQ Write File 2"("error in (no error)"=w328, "Image Quality"=u32 1000, "File Path"=w351, "Image"=w329) -> ("error out"=w343:errorcluster)  [unwired: 6 in, 1 out]
            n116 = Path To String(path=w339) -> (string=w337:string)
            n117 = Path To String(path=w338) -> (string=w336:string)
            n118 = local read "Command File Location"() -> (w340:path)
            n119 = Bundle By Name(cluster=T6 {"Source"="", "Destination"="", "CMD"="newfolders", "Time"="time"} ("Output JSON File"), "Source"=w337, "Destination"=w336, "CMD"="restart") -> (w345:T6)
            n120 = Flatten To JSON(anything=w345, error in (no error)=w343) -> (JSON string=w346:string, 11:w342:errorcluster)  [unwired: 1 in]
            n121 = Write to Text File(file (use dialog)=w340, text=w346, error in=w342) -> (error out=w322:errorcluster)  [unwired: 1 in, 2 out]
            n122 = local write "Play Button"(w320) -> ()
            n123 = local write "Calibrate"(w320) -> ()
            n124 = local write "Pause Button"(w320) -> ()
            n125 = local write "Save Button"(w320) -> ()
            n126 = property on="Play Button" class="Bool (strict)"("DisabledEnum"=T4."Enabled" ("Disabled")) -> ()  [unwired: 2 in, 2 out]
          }
          event "Play Button": Value Change {
            w362 = T4."Disabled and Grayed Out" ("Disabled")
            # "Log Imaging Params"
            # "Enable the pause button"
            # "Disable all controls on the front panel except the pause button"
            n127 = event-data() -> ()  [unwired: 1 in, 3 out]
            n128 = property on="Pause Button" class="Bool (strict)"("DisabledEnum"=T4."Enabled" ("Disabled")) -> ()  [unwired: 2 in, 2 out]
            n129 = property on="Play Button" class="Bool (strict)"("DisabledEnum"=w362) -> ()  [unwired: 2 in, 2 out]
            n130 = property on="HRME Exposure" class="Slide (strict)"("DisabledEnum"=w362) -> ()  [unwired: 2 in, 2 out]
            n131 = property on="Calibrate" class="Bool (strict)"("DisabledEnum"=w362) -> ()  [unwired: 2 in, 2 out]
            n132 = property on="HRME Gain" class="Slide (strict)"("DisabledEnum"=w362) -> ()  [unwired: 2 in, 2 out]
            n133 = local write "Pause Button"(FALSE) -> ()
            n134 = property on="Close Program" class="Bool (strict)"("DisabledEnum"=w362) -> ()  [unwired: 2 in, 2 out]
            n135 = property on="Auto Gain" class="Bool (strict)"("DisabledEnum"=w362) -> ()  [unwired: 2 in, 2 out]
            n136 = property on="Save Button" class="Bool (strict)"("DisabledEnum"=w362) -> ()  [unwired: 2 in, 2 out]
            n137 = property on="Auto Exposure" class="Bool (strict)"("DisabledEnum"=w362) -> ()  [unwired: 2 in, 2 out]
            n138 = local read "Auto Exposure"() -> (w365:bool)
            n139 = local read "Auto Gain"() -> (w366:bool)
            n140 = local read "HRME Exposure"() -> (w367:dbl)
            n141 = local read "HRME Gain"() -> (w368:dbl)
            n142 = local read "Log File Out"() -> (w369:refnum<file>)
            n143 = call "Esophageal_Datalogger_PlayButton.vi"("Gain Value"=w368, "Auto Exposure Status"=w365, "error in (no error)"=w361, "Exposure Value"=w367, "Auto Gain Status"=w366, "Log File In"=w369) -> ("error out"=w364:errorcluster)  [unwired: 4 in, 1 out]
          }
          event "Auto Gain": Value Change {
            # "Might have to come back to this one....we'll have to wait and see"
            # "Disable if autogain is turned on"
            # "Select on/off"
            # "Turn auto gain on or off"
            n144 = event-data() -> ("NewVal"=w379:bool)  [unwired: 1 in, 2 out]
            n145 = Select(t=u32 1 ("ValueU32"), s=w379, f=u32 0 ("ValueU32")) -> (s? t:f=w382:u32)
            n146 = Select(t=T4."Disabled and Grayed Out" ("Disabled"), s=w379, f=T4."Enabled" ("Disabled")) -> (s? t:f=w378:T4)
            n147 = property class="IMAQdx"(reference=w388, error in=w386, "ActiveAttribute"="CameraAttributes::AnalogControl::GainAuto", "ValueU32"=w382) -> (reference out=w387:T8, error out=w377:errorcluster)
            n148 = property on="HRME Gain" class="Slide (strict)"(error in=w377, "DisabledEnum"=w378) -> (error out=w376:errorcluster)  [unwired: 1 in, 1 out]
          }
          event "Auto Exposure": Value Change {
            # "this is another one we'll probably have to come back to"
            # "Disable if autogain is turned on"
            n149 = event-data() -> ("NewVal"=w392:bool)  [unwired: 1 in, 2 out]
            n150 = Select(t=u32 1 ("ValueU32"), s=w392, f=u32 0 ("ValueU32")) -> (s? t:f=w404:u32)
            n151 = Select(t=T4."Disabled and Grayed Out" ("Disabled"), s=w392, f=T4."Enabled" ("Disabled")) -> (s? t:f=w393:T4)
            n152 = property class="IMAQdx"(reference=w401, error in=w399, "ActiveAttribute"="CameraAttributes::AcquisitionControl::ExposureAuto", "ValueU32"=w404) -> (reference out=w400:T8, error out=w395:errorcluster)
            n153 = property on="HRME Exposure" class="Slide (strict)"(error in=w395, "DisabledEnum"=w393) -> (error out=w394:errorcluster)  [unwired: 1 in, 1 out]
          }
          event "Close Program": Value Change {
            n154 = event-data() -> ()  [unwired: 1 in, 3 out]
            n155 = local write "Close Program"(FALSE) -> ()
          }
          event "HRME Exposure": Value Change {
            # "Change fastHRME Exposure"
            n156 = event-data() -> ()  [unwired: 1 in, 6 out]
            n157 = property class="IMAQdx"(reference=w417, error in=w413, "ActiveAttribute"="CameraAttributes::AcquisitionControl::ExposureTime", "ValueU32"="HRME Exposure") -> (reference out=w416:T8, error out=w412:errorcluster)
          }
          event "HRME Gain": Value Change {
            # "Change fastHRME Gain"
            n158 = event-data() -> ()  [unwired: 1 in, 6 out]
            n159 = property class="IMAQdx"(reference=w426, error in=w423, "ActiveAttribute"="CameraAttributes::AnalogControl::Gain", "ValueU32"="HRME Gain") -> (reference out=w425:T8, error out=w424:errorcluster)
          }
          event "Save Button": Value Change {
            w466 = u32 1 items=["Frame", "Fill", "Highlight"] ("Drawing Mode (Frame)")
            w482 = T11 0 items=["Grayscale (U8)", "Grayscale (I16)", "Grayscale (SGL)", "Complex (CSG)", "RGB (U32)", "HSL (U32)", "RGB (U64)", "Grayscale (U16)"] ("Image Type")
            # "location of python file"
            # "creat json file path 2 save img score"
            # "Log Image Params"
            # "Overlay Colored Box"
            # "Cast to External Monitor"
            # "Update Number of Images Acquired"
            # "Generate Filename"
            # "Acquire Image"
            # "Get Exposure and Gain Values"
            # "Save Image to File"
            n160 = event-data() -> ()  [unwired: 1 in, 6 out]
            n161 = local read "Saved Imaged Number"() -> (w484:i32)
            n162 = local write "Save Button"(FALSE) -> ()
            n163 = property class="IMAQdx"(reference=w478, "ActiveAttribute"="CameraAttributes::AcquisitionControl::ExposureTime", "ActiveAttribute"="CameraAttributes::AnalogControl::Gain") -> (reference out=w488:T8, "ValueU32"=w487:u32, "ValueU32"=w486:u32)  [unwired: 1 in, 1 out]
            n164 = call "IMAQ Cast Image 2"("Image Src"=w477, "Image Type"=w482, "error in (no error)"=w476) -> ("Image Dst Out"=w481:T1, "error out"=w480:errorcluster)  [unwired: 11 in]
            n165 = local read "Representative Images"() -> (w451:path)
            n166 = Increment(x=w484) -> (x+1=w459:i32)
            n167 = call "Esophageal_Generate_Image_Filename.vi"("Image Number"=w459, "HRME Gain"=w486, "HRME Exposure"=w487) -> ("Notification Text"=→"Image Save Notification":string, "Image Filename"=w452:string)  [unwired: 7 in]
            n168 = Build Path(base path=w451, name or relative path=w452) -> (appended path=w493:path)
            n169 = property class="Enum (strict)"(reference=w460) -> ("Value"=w461:enum16{"15.9", "24.0"})  [unwired: 1 in, 2 out]
            n170 = local write "Saved Imaged Number"(w459) -> ()
            n171 = call-poly "IMAQ Write File 2"("error in (no error)"=w480, "Image Quality"=u32 1000, "File Path"=w493, "Image"=w481) -> ("error out"=w444:errorcluster, "Image Out (duplicate)"=w491:T1)  [unwired: 6 in]
            n172 = case shown="\"15.9\", Default" w461 {
              tunnel: [15.9 24.0] -> w436
              frame "15.9", Default {
              }
              frame "24.0" {
              }
            }
            n173 = Build Path(base path=w451, name or relative path=w452) -> (appended path=w453:path)
            n174 = Search/Split String(string=w452, search string/char (-)=".") -> (substring before match=w456:string)  [unwired: 1 in, 2 out]
            n175 = Path To String(path=w453) -> (string=w447:string)
            n176 = Concatenate Strings(w456, ".json") -> (w455:string)
            n177 = local read "HRME Scores"() -> (w450:path)
            n178 = property on="Image Analysis Meter" class="Slide (strict)"("DisabledEnum"=T4."Enabled" ("Disabled")) -> ()  [unwired: 2 in, 2 out]
            n179 = Build Path(base path=path "C:/Users/EsophaHRME_Dell2/Documents/GitHub/Esophageal_HRME_Software/EsophagealDeployment/Multi_Task_Network", name or relative path="score_rep_img.py") -> (appended path=w445:path)
            n180 = Build Path(base path=w450, name or relative path=w455) -> (appended path=w454:path)
            n181 = Path To String(path=w454) -> (string=w441:string)
            n182 = node(w446, w445, "process_single_image", w444, "", w447, w441) -> (w430:refnum<k35>, w431:errorcluster, w432:string)  [unwired: 2 in, 2 out]
            n183 = Fract/Exp String To Number(string=w432) -> (number=w437:dbl)  [unwired: 3 in, 1 out]
            n184 = Multiply(x=w437, y=100.0) -> (x*y=w434:dbl)
            "Image Analysis Meter" <- w434
            n185 = Greater?(x=w434, y=w436) -> (0:w440:bool)
            n186 = Select(t=u32 16718848, s=w440, f=u32 65289) -> (s? t:f=w433:u32)
            n187 = property on="Image Analysis Meter" class="Slide (strict)"(error in=w431, "Fill Color"=w433) -> (error out=w464:errorcluster)  [unwired: 1 in, 1 out]
            n188 = local read "Timestamp"() -> (w465:string)
            n189 = local read "Log File Out"() -> (w462:refnum<file>)
            n190 = local read "HRME Image"() -> (w472:T1)
            n191 = call "Esophageal_Datalogger_SaveButton.vi"("HRME Score"=w432, "error in (no error)"=w464, "Timestamp"=w465, "Image Name"=w452, "Log File In"=w462) -> ("error out"=w463:errorcluster)  [unwired: 5 in, 1 out]
            n192 = call "IMAQ Overlay Rectangle"("Color"=w433, "Group"=w432, "error in (no error)"=w463, "Drawing Mode (Frame)"=w466, "Rectangle"=T7 {"Left"=0, "Top"=0, "Right"=50, "Bottom"=50}, "Image"=w472) -> ("error out"=w468:errorcluster, "Image Out"=w471:T1)  [unwired: 4 in]
            n193 = local read "Height"() -> (w475:i16)
            n194 = call "IMAQ Merge Overlay"("error in (no error)"=w468, "Image Src"=w471) -> ("error out"=w469:errorcluster, "Image Dst Out"=w470:T1)  [unwired: 8 in]
            n195 = local read "Width"() -> (w474:i16)
            n196 = call "Esophageal_CastImage.vi"("X Resolution"=w474, "Y Resolution"=w475, "error in (no error)"=w469, "Image In"=w470) -> ("error out"=w473:errorcluster)  [unwired: 7 in]
          }
        }
        n197 = local write "Recording"(FALSE ("Recording")) -> ()
        n198 = call <extravilib>:"Read.vi"("channel"=w138) -> ("element"=w137:bool)  [unwired: 1 in, 1 out]
        n199 = case shown="False" w137 {
          selector: w137 -> [w266 _]
          tunnel: w141 -> [w267 w281]
          tunnel: [w267 w280] -> w168
          tunnel: [w266 w279] -> w167
          tunnel: w140 -> [w265 w278]
          tunnel: [w265 w268] -> w164
          frame False {
          }
          frame True {
            w277 = T4."Disabled and Grayed Out" ("Disabled")
            # "Log Imaging Params"
            # "Enable the pause button"
            # "Disable all controls on the front panel except the pause button"
            # "Waits until the foot pedal is done being pressed."
            n200 = while {
              tunnel: w281 -> [w289]
              tunnel: [w288] -> w280
              tunnel: [w284] -> w279
              tunnel: w278 -> [w285]
              tunnel: [w282] -> w275
              stop <- w283 stop-if-true
              n201 = call-poly <vilib>:"DAQmx Read.vi"("task/channels in"=w289, "error in"=w285) -> ("task out"=w288:refnum<k21>, "data"=w286:bool[], "error out"=w282:errorcluster)  [unwired: 11 in]
              n202 = Index Array(array=w286, index=0) -> (element=w284:bool)
              n203 = Or(x=w284, y=w282) -> (x .or. y?=w283:bool)
            }
            n204 = property on="Play Button" class="Bool (strict)"("DisabledEnum"=w277) -> ()  [unwired: 2 in, 2 out]
            n205 = property on="Calibrate" class="Bool (strict)"("DisabledEnum"=w277) -> ()  [unwired: 2 in, 2 out]
            n206 = property on="Close Program" class="Bool (strict)"("DisabledEnum"=w277) -> ()  [unwired: 2 in, 2 out]
            n207 = property on="Save Button" class="Bool (strict)"("DisabledEnum"=w277) -> ()  [unwired: 2 in, 2 out]
            n208 = property on="HRME Exposure" class="Slide (strict)"("DisabledEnum"=w277) -> ()  [unwired: 2 in, 2 out]
            n209 = property on="HRME Gain" class="Slide (strict)"("DisabledEnum"=w277) -> ()  [unwired: 2 in, 2 out]
            n210 = property on="Pause Button" class="Bool (strict)"(error in=w275, "DisabledEnum"=T4."Enabled" ("Disabled")) -> (error out=w269:errorcluster)  [unwired: 1 in, 1 out]
            n211 = property on="Auto Gain" class="Bool (strict)"("DisabledEnum"=w277) -> ()  [unwired: 2 in, 2 out]
            n212 = property on="Auto Exposure" class="Bool (strict)"("DisabledEnum"=w277) -> ()  [unwired: 2 in, 2 out]
            n213 = local read "Auto Exposure"() -> (w270:bool)
            n214 = local read "Auto Gain"() -> (w271:bool)
            n215 = local read "HRME Exposure"() -> (w272:dbl)
            n216 = local read "HRME Gain"() -> (w273:dbl)
            n217 = local read "Log File Out"() -> (w274:refnum<file>)
            n218 = call "Esophageal_Datalogger_PlayButton.vi"("Gain Value"=w273, "Auto Exposure Status"=w270, "error in (no error)"=w269, "Exposure Value"=w272, "Auto Gain Status"=w271, "Log File In"=w274) -> ("error out"=w268:errorcluster)  [unwired: 4 in, 1 out]
          }
        }
        n219 = while {
          shift-right: [w243] -> _
          shift-left: w147 -> [w242]
          shift-right: [w237] -> _
          shift-left: w146 -> [w241]
          shift-right: [w234] -> w148
          shift-left: w149 -> [w240]
          tunnel: [w239] -> w155
          tunnel: [w238] -> w154
          tunnel: w151 -> [w225]
          tunnel: w150 -> [w224]
          tunnel: w145 -> [w220]
          tunnel: w144 -> [w217]
          tunnel: w139 -> [w214]
          i -> [w231]
          stop <- w211 stop-if-true
          # "Attempt to slow down frame rate"
          n220 = call <vilib>:"IMAQdx Grab2.vi"("error in"=w240, "Image In"=w241, "Session In"=w242) -> ("error out"=w236:errorcluster, "Image Out"=w237:T1, "Session Out"=w243:T8)  [unwired: 5 in, 1 out]
          n221 = call <extravilib>:"Read.vi"("channel"=w224) -> ("element"=w223:bool)  [unwired: 1 in, 1 out]
          n222 = call <extravilib>:"Read.vi"("channel"=w225) -> ("element"=w222:bool)  [unwired: 1 in, 1 out]
          n223 = call <extravilib>:"Read.vi"("channel"=w220) -> ("element"=w219:bool)  [unwired: 1 in, 1 out]
          n224 = Quotient & Remainder(x=w231, y=4) -> (x-y*floor(x/y)=w229:i32)  [unwired: 1 out]
          n225 = call <extravilib>:"Read.vi"("channel"=w217) -> ("element"=w216:bool)  [unwired: 1 in, 1 out]
          n226 = Equal To 0?(x=w229) -> (x = 0?=w226:bool)
          n227 = call <extravilib>:"Read.vi"("channel"=w214) -> ("element"=w213:bool)  [unwired: 1 in, 1 out]
          n228 = Or(x=w226, y=TRUE) -> (x .or. y?=w228:bool)
          n229 = call "IMAQ Resample"("X Resolution"=960, "Y Resolution"=540, "error in (no error)"=w236, "Image Src"=w237) -> ("error out"=w235:errorcluster, "Image Dst Out"=w221:T1)  [unwired: 6 in]
          n230 = Or(x=w223, y=w222) -> (x .or. y?=w218:bool)
          n231 = Or(x=w218, y=w219) -> (x .or. y?=w215:bool)
          n232 = Or(x=w215, y=w216) -> (x .or. y?=w212:bool)
          n233 = Or(x=w213, y=w212) -> (x .or. y?=w211:bool)
          n234 = case shown="True" w228 {
            tunnel: [_ w254] -> w239
            tunnel: [_ w249] -> w238
            tunnel: w211 -> [_ w245]
            tunnel: w235 -> [w244 w248]
            tunnel: [w244 w247] -> w234
            tunnel: w221 -> [_ w246]
            frame False {
            }
            frame True {
              n235 = Format Date/Time String(time format string (%c)="%H%M%S%3u") -> (date/time string=w251:string)  [unwired: 2 in]
              n236 = call "IMAQ ColorImageToArray"("Image"=w246, "error in (no error)"=w248) -> ("Image Pixels (U32)"=w255:u32[][], "error out"=w247:errorcluster)  [unwired: 2 in, 1 out]
              n237 = Concatenate Strings(w251, ".png" ("string")) -> (w250:string)
              n238 = call <extravilib>:"Write.vi"("last element? (F)"=w245, "element"=w255) -> ("channel"=w254:T14)  [unwired: 7 in, 2 out]
              n239 = call <extravilib>:"Write.vi"("last element? (F)"=w245, "element"=w250) -> ("channel"=w249:T15)  [unwired: 7 in, 2 out]
            }
          }
        }
        n240 = call "IMAQ Create"("Image Name"="Endoscope Consumer", "Image Type"=w152) -> ("New Image"=w153:T1)  [unwired: 3 in, 1 out]
        n241 = while {
          tunnel: w155 -> [w210]
          tunnel: w154 -> [w209]
          shift-right: [w203] -> _
          shift-left: w153 -> [w207]
          stop <- w201 stop-if-true
          # "Take filename from channel"
          # "Take image from channel"
          # "Save the image to file"
          # "Reads image from channel, converts it into an image, then writes that image to file."
          n242 = local read "WideField Path"() -> (w200:path)
          n243 = call <extravilib>:"Read.vi"("channel"=w209) -> ("element"=w206:string)  [unwired: 6 in, 4 out]
          n244 = call <extravilib>:"Read.vi"("channel"=w210) -> ("done?"=w201:bool, "element"=w208:u32[][])  [unwired: 6 in, 3 out]
          n245 = call "IMAQ ArrayToColorImage"("Image Pixels (U32)"=w208, "Image"=w207) -> ("Image Out"=w204:T1)  [unwired: 3 in, 1 out]
          n246 = Build Path(base path=w200, name or relative path=w206) -> (appended path=w202:path)
          n247 = call-poly "IMAQ Write File 2"("Image Quality"=u32 1000, "File Path"=w202, "Image"=w204) -> ("Image Out (duplicate)"=w203:T1)  [unwired: 7 in, 1 out]
        }
        n248 = Select(t=Esophogeal_Software_States."Imaging" ("Anal HRME States"), s=w167, f=w171) -> (s? t:f=w172:T2)
        n249 = Merge Errors(w163, w164, w161) -> (w162:errorcluster)
      }
      frame "Imaging" {
        w506 = T11 4 items=["Grayscale (U8)", "Grayscale (I16)", "Grayscale (SGL)", "Complex (CSG)", "RGB (U32)", "HSL (U32)", "RGB (U64)", "Grayscale (U16)"] ("Image Type")
        # "Log Imaging Paused"
        # "Turn Red Light on to indicate frames are now being saved"
        n250 = while {
          tunnel: w523 -> [w613]
          tunnel: w522 -> [w612]
          tunnel: [w581] -> w521
          tunnel: [w591] -> w520
          tunnel: [w608] -> w504
          tunnel: w505 -> [w610]
          shift-right: [w605] -> w516
          shift-left: w519 -> [w611]
          tunnel: [w604] -> w515
          tunnel: [w602] -> w512
          tunnel: [w582] -> w507
          tunnel: [w580] -> w501
          stop <- w603 stop-if-true
          w588 = T4."Disabled and Grayed Out" ("Disabled")
          w589 = T11 0 items=["Grayscale (U8)", "Grayscale (I16)", "Grayscale (SGL)", "Complex (CSG)", "RGB (U32)", "HSL (U32)", "RGB (U64)", "Grayscale (U16)"] ("Image Type")
          # "Converts image to array"
          # "Generate filename from timestamp"
          # "Send to producer"
          # "Read Foot Pedal Status"
          # "Acquire fastHRME Image"
          n251 = call <vilib>:"IMAQdx Grab2.vi"("error in"=w610, "Image In"=w612, "Session In"=w613) -> ("error out"=w590:errorcluster, "Image Out"=w591:T1, "Session Out"=w581:T8)  [unwired: 5 in, 1 out]
          n252 = call "IMAQ Cast Image 2"("Image Src"=w591, "Image Type"=w589, "error in (no error)"=w590) -> ("Image Dst Out"=w585:T1, "error out"=w584:errorcluster)  [unwired: 11 in]
          n253 = local read "Height"() -> (w587:i16)
          n254 = local write "HRME Image"(w585) -> ()
          n255 = Format Date/Time String(time format string (%c)="%H%M%S%3u") -> (date/time string=w594:string)  [unwired: 2 in]
          n256 = local read "Width"() -> (w586:i16)
          n257 = call "IMAQ ImageToArray"("Image"=w585) -> ("Image Pixels (U8)"=w595:u8[][])  [unwired: 3 in, 4 out]
          n258 = call-poly <vilib>:"DAQmx Read.vi"("task/channels in"=w611, "error in"=w610) -> ("task out"=w597:refnum<k21>, "data"=w599:bool[], "error out"=w596:errorcluster)  [unwired: 11 in]
          n259 = call "Esophageal_CastImage.vi"("X Resolution"=w586, "Y Resolution"=w587, "error in (no error)"=w584, "Image In"=w585) -> ("error out"=w583:errorcluster)  [unwired: 7 in]
          n260 = Concatenate Strings(w594, ".png" ("string")) -> (w580:string)
          n261 = call <extravilib>:"Write.vi"("element"=w580) -> ("channel"=w602:T15)  [unwired: 8 in, 2 out]
          n262 = Index Array(array=w599, index=0) -> (element=w600:bool)
          n263 = Not(x=w600) -> (.not. x?=w598:bool)
          n264 = case shown="True" w598 {
            selector: w598 -> [w615 _]
            tunnel: w597 -> [w616 w621]
            tunnel: [w616 w620] -> w605
            tunnel: [w615 w617] -> w606
            tunnel: w596 -> [w614 w619]
            tunnel: [w614 w618] -> w609
            frame False {
            }
            frame True {
              # "Waits until the foot pedal is done being pressed."
              n265 = while {
                tunnel: w621 -> [w628]
                tunnel: [w627] -> w620
                tunnel: [w624] -> w617
                tunnel: w619 -> [w623]
                tunnel: [w622] -> w618
                stop <- w624 stop-if-true
                n266 = call-poly <vilib>:"DAQmx Read.vi"("task/channels in"=w628, "error in"=w623) -> ("task out"=w627:refnum<k21>, "data"=w625:bool[], "error out"=w622:errorcluster)  [unwired: 11 in]
                n267 = Index Array(array=w625, index=0) -> (element=w624:bool)
              }
            }
          }
          n268 = property on="Save Button" class="Bool (strict)"("DisabledEnum"=w588) -> ()  [unwired: 2 in, 2 out]
          n269 = property on="Play Button" class="Bool (strict)"("DisabledEnum"=w588) -> ()  [unwired: 2 in, 2 out]
          n270 = property on="Image Analysis Meter" class="Slide (strict)"("DisabledEnum"=w588) -> ()  [unwired: 2 in, 2 out]
          n271 = Or(x="Pause Button", y=w606) -> (x .or. y?=w603:bool)
          "Pause Status" <- w603
          n272 = call <extravilib>:"Write.vi"("last element? (F)"=w603, "element"=w595) -> ("channel"=w604:T16)  [unwired: 7 in, 2 out]
          n273 = Merge Errors(w583, w609) -> (w608:errorcluster)
          n274 = call <extravilib>:"Write.vi"("element"=w603) -> ("channel"=w582:T12)  [unwired: 1 out]
        }
        "Timestamp" <- w501
        n275 = while {
          shift-right: [w556] -> _
          shift-left: w499 -> [w555]
          shift-right: [w549] -> _
          shift-left: w498 -> [w554]
          shift-right: [w546] -> w497
          shift-left: w500 -> [w553]
          tunnel: [w552] -> w510
          tunnel: [w551] -> w509
          tunnel: w507 -> [w550]
          i -> [w542]
          stop <- w539 stop-if-true
          # "Attempt to slow down frame rate"
          n276 = call <vilib>:"IMAQdx Grab2.vi"("error in"=w553, "Image In"=w554, "Session In"=w555) -> ("error out"=w548:errorcluster, "Image Out"=w549:T1, "Session Out"=w556:T8)  [unwired: 5 in, 1 out]
          n277 = call <extravilib>:"Read.vi"("channel"=w550) -> ("element"=w539:bool)  [unwired: 1 in, 1 out]
          n278 = Quotient & Remainder(x=w542, y=4) -> (x-y*floor(x/y)=w540:i32)  [unwired: 1 out]
          n279 = Equal To 0?(x=w540) -> (x = 0?=w538:bool)
          n280 = Or(x=w538, y=w539) -> (x .or. y?=w537:bool)
          n281 = call "IMAQ Resample"("X Resolution"=960, "Y Resolution"=540, "error in (no error)"=w548, "Image Src"=w549) -> ("error out"=w547:errorcluster, "Image Dst Out"=w545:T1)  [unwired: 6 in]
          "Endoscope Feed" <- w545
          n282 = case shown="True" w537 {
            tunnel: [_ w567] -> w552
            tunnel: [_ w562] -> w551
            tunnel: w539 -> [_ w558]
            tunnel: w547 -> [w557 w561]
            tunnel: [w557 w560] -> w546
            tunnel: w545 -> [_ w559]
            frame False {
            }
            frame True {
              n283 = Format Date/Time String(time format string (%c)="%H%M%S%3u") -> (date/time string=w564:string)  [unwired: 2 in]
              n284 = call "IMAQ ColorImageToArray"("Image"=w559, "error in (no error)"=w561) -> ("Image Pixels (U32)"=w568:u32[][], "error out"=w560:errorcluster)  [unwired: 2 in, 1 out]
              n285 = Concatenate Strings(w564, ".png" ("string")) -> (w563:string)
              n286 = call <extravilib>:"Write.vi"("last element? (F)"=w558, "element"=w568) -> ("channel"=w567:T14)  [unwired: 7 in, 2 out]
              n287 = call <extravilib>:"Write.vi"("last element? (F)"=w558, "element"=w563) -> ("channel"=w562:T15)  [unwired: 7 in, 2 out]
            }
          }
        }
        n288 = call "IMAQ Create"("Image Name"="Endoscope Consumer", "Image Type"=w506) -> ("New Image"=w508:T1)  [unwired: 3 in, 1 out]
        n289 = call "IMAQ Create"("Image Name"="HRME Consumer") -> ("New Image"=w513:T1)  [unwired: 4 in, 1 out]
        n290 = while {
          tunnel: w510 -> [w536]
          tunnel: w509 -> [w535]
          shift-right: [w528] -> _
          shift-left: w508 -> [w533]
          stop <- w526 stop-if-true
          # "Take filename from channel"
          # "Take image from channel"
          # "Save the image to file"
          # "Reads image from channel, converts it into an image, then writes that image to file."
          n291 = local read "WideField Path"() -> (w532:path)
          n292 = call <extravilib>:"Read.vi"("channel"=w536) -> ("done?"=w526:bool, "element"=w534:u32[][])  [unwired: 6 in, 3 out]
          n293 = call <extravilib>:"Read.vi"("channel"=w535) -> ("element"=w531:string)  [unwired: 6 in, 4 out]
          n294 = call "IMAQ ArrayToColorImage"("Image Pixels (U32)"=w534, "Image"=w533) -> ("Image Out"=w529:T1)  [unwired: 3 in, 1 out]
          n295 = Build Path(base path=w532, name or relative path=w531) -> (appended path=w527:path)
          n296 = call-poly "IMAQ Write File 2"("Image Quality"=u32 1000, "File Path"=w527, "Image"=w529) -> ("Image Out (duplicate)"=w528:T1)  [unwired: 7 in, 1 out]
        }
        n297 = while {
          tunnel: w515 -> [w579]
          shift-right: [w575] -> _
          shift-left: w513 -> [w571]
          tunnel: w512 -> [w574]
          stop <- w578 stop-if-true
          # "Reads image from channel, converts it into an image, then writes that image to file."
          n298 = local read "HRME Path"() -> (w570:path)
          n299 = call <extravilib>:"Read.vi"("channel"=w579) -> ("done?"=w578:bool, "element"=w577:u8[][])  [unwired: 6 in, 3 out]
          n300 = call <extravilib>:"Read.vi"("channel"=w574) -> ("element"=w572:string)  [unwired: 6 in, 4 out]
          n301 = call "IMAQ ArrayToImage"("Image Pixels (U8)"=w577, "Image"=w571) -> ("Image Out"=w576:T1)  [unwired: 8 in, 1 out]
          n302 = Build Path(base path=w570, name or relative path=w572) -> (appended path=w573:path)
          n303 = call-poly "IMAQ Write File 2"("Image Quality"=u32 1000, "File Path"=w573, "Image"=w576) -> ("Image Out (duplicate)"=w575:T1)  [unwired: 7 in, 1 out]
        }
        n304 = local read "Log File Out"() -> (w502:refnum<file>)
        n305 = call "Esophageal_Datalogger_PauseButton.vi"("error in (no error)"=w504, "Log File In"=w502) -> ("error out"=w503:errorcluster)  [unwired: 8 in, 1 out]
        "Recording" <- TRUE ("Recording")
      }
      frame "Endo Only Saving" {
        w629 = FALSE
        w630 = T4."Enabled" ("Disabled")
        w631 = T4."Disabled and Grayed Out" ("Disabled")
        w647 = T11 4 items=["Grayscale (U8)", "Grayscale (I16)", "Grayscale (SGL)", "Complex (CSG)", "RGB (U32)", "HSL (U32)", "RGB (U64)", "Grayscale (U16)"] ("Image Type")
        # "Just realized that we probably don't have to come back here after calibrate is clicked. Instead we can stay in the image prep section. \nHere we can keep collecting the endo frames by being in the time out section. When the calibrate button is clicked it turns off the \nwhile loop collecting the endo frames and does what it needs to do. Then it goes back to time out. Form here you can click whatever\nyou want. It might work better than having to back here.\n\nSo we don't have to implement the turning off the while loop if the play button is clicked. We again also don't ever have to come back\nhere hopefully."
        # "We reach this state right form the start of the program. We want to be collecting endo frames the whole time while \nnot having to collect HRME frames. This state allows us to do that.  After the initialize state we come to this state. \n\nWe come in here start collecting endo frames and can only leave this state when the user clicks calibrate, play , or close program. \nSince this is the first place we go to it means we havne't calibrated the HRME yet.  So we have to do that at some point. \nClick calibrate and then take us there and the calibrationwill happen automatically. We then get take back here from calibrate. \nWe restart collecting endo frames but maybe it's moved fast enough that it wasn't noticed. (WE'll HAVE TO SEE HOW FAST THE\nDELAY IS). This doesn't mean that the callibration was good though so the button can still be clicked and repeat the process. \n\nIf the calibration was good enough that means we either wnat to continue collecting endo images only, start collecting HRME, \nor close the program. For the first part we don't have to do anything. To start collecting HRME images, we can hit play and from\nthere on we don't have to come back to this state again. Close program will obviously turn off everything. \n\nSo with this in mind we have to get out of the while loop when either the close porgram, calibrate, or play buttons are clicked.\nI haven't found a way to check on the button status without a boolean status flag like the 'pause status'. I don't know how to \nimplement that so instead I have the local variables created from the buttons. From what I'm able to tell, they're always being \nchecked and when they are changed the first while loop lets the endo loop know that it needs to stop. WIll this cause problems?\nI have not idea right now. But either way I'll run through the steps that I think are being taken and some explanations. \n\nSteps that are followed by the flow...hopefully:\n\n1. Turn off all buttons ( Needs to happen because the buttons have been changed from mechanical action latch to switch) \n2. Turn on calibrate and close program ( These are the only two buttons that will allow you to leave this state)\n3. This might be weird. I don't know if the while loop checking the buttons statuses happens first or if it happens after the endo\n     loop. I'll leave it here for now but depending on when it starts it could break some things. Either way this while loop starts\n     checking for the button statuses.\n4. The endo scrope start collecting the frames. The loop will only break when one of the buttons has been clicked. If the butotn is \n     clicked it also means that it is the last element which is why we're passing that true vlaue to the case block within the loop. The\n     frame rate might mess some things up but we'll know that when we get there. Either way it is alwasy checking for the \n     remainder and if it's 0 then we can save an image. If it's not then we wait till it is.\n5. The image that is collected from the endo frame while is passed into the save endo while loop. Here we just save the endo \n     frame. I think it turns off when the image is saved. So it doens't really get stuck in an infinite loop here.\n6. Turn off the calibrate and close program buttons then immediately turn them back on. This resets them since we moved\n     from latch mechanical action to switch. Which means that the buttons stays in the state that the user left it in. So click and it\n     stays clicked. Unclick and it stays unclicked. The latch mechanism had it working so that when you click it unclicks itself."
        n306 = property on="Close Program" class="Bool (strict)"("DisabledEnum"=w630) -> ()  [unwired: 2 in, 2 out]
        n307 = property on="Calibrate" class="Bool (strict)"("DisabledEnum"=w630) -> ()  [unwired: 2 in, 2 out]
        n308 = property on="Save Button" class="Bool (strict)"("DisabledEnum"=w631) -> ()  [unwired: 2 in, 2 out]
        n309 = property on="Auto Gain" class="Bool (strict)"("DisabledEnum"=w631) -> ()  [unwired: 2 in, 2 out]
        n310 = property on="HRME Gain" class="Slide (strict)"("DisabledEnum"=w631) -> ()  [unwired: 2 in, 2 out]
        n311 = property on="Pause Button" class="Bool (strict)"("DisabledEnum"=w631) -> ()  [unwired: 2 in, 2 out]
        n312 = property on="Auto Exposure" class="Bool (strict)"("DisabledEnum"=w631) -> ()  [unwired: 2 in, 2 out]
        n313 = property on="HRME Exposure" class="Slide (strict)"("DisabledEnum"=w631) -> ()  [unwired: 2 in, 2 out]
        n314 = while {
          tunnel: [w676] -> w636
          tunnel: [w675] -> w635
          stop <- w672 stop-if-true
          n315 = local read "Calibrate"() -> (w674:bool)
          n316 = call <extravilib>:"Write.vi"("element"=w674) -> ("channel"=w676:T12)  [unwired: 1 out]
          n317 = local read "Close Program"() -> (w673:bool)
          n318 = call <extravilib>:"Write.vi"("element"=w673) -> ("channel"=w675:T12)  [unwired: 1 out]
          n319 = Or(x=w674, y=w673) -> (x .or. y?=w672:bool)
        }
        n320 = while {
          tunnel: [w667] -> w639
          tunnel: [w671] -> w638
          tunnel: [w659] -> w637
          tunnel: w642 -> [w666]
          tunnel: w641 -> [w665]
          tunnel: w640 -> [w664]
          tunnel: w636 -> [w658]
          tunnel: w635 -> [w657]
          stop <- w654 stop-if-true
          w660 = T4."Disabled and Grayed Out" ("Disabled")
          w669 = T11 0 items=["Grayscale (U8)", "Grayscale (I16)", "Grayscale (SGL)", "Complex (CSG)", "RGB (U32)", "HSL (U32)", "RGB (U64)", "Grayscale (U16)"] ("Image Type")
          # "Acquire fastHRME Image"
          n321 = call <vilib>:"IMAQdx Grab2.vi"("error in"=w664, "Image In"=w665, "Session In"=w666) -> ("error out"=w670:errorcluster, "Image Out"=w671:T1, "Session Out"=w667:T8)  [unwired: 5 in, 1 out]
          n322 = call <extravilib>:"Read.vi"("channel"=w658) -> ("element"=w656:bool)  [unwired: 1 in, 1 out]
          n323 = call <extravilib>:"Read.vi"("channel"=w657) -> ("element"=w655:bool)  [unwired: 1 in, 1 out]
          n324 = Or(x=w656, y=w655) -> (x .or. y?=w654:bool)
          n325 = call "IMAQ Cast Image 2"("Image Src"=w671, "Image Type"=w669, "error in (no error)"=w670) -> ("Image Dst Out"=w663:T1, "error out"=w668:errorcluster)  [unwired: 11 in]
          n326 = local write "HRME Image"(w663) -> ()
          n327 = property on="Save Button" class="Bool (strict)"("DisabledEnum"=w660) -> ()  [unwired: 2 in, 2 out]
          n328 = local read "Height"() -> (w662:i16)
          n329 = local read "Width"() -> (w661:i16)
          n330 = call "Esophageal_CastImage.vi"("X Resolution"=w661, "Y Resolution"=w662, "error in (no error)"=w668, "Image In"=w663) -> ("error out"=w659:errorcluster)  [unwired: 7 in]
          n331 = property on="Image Analysis Meter" class="Slide (strict)"("DisabledEnum"=w660) -> ()  [unwired: 2 in, 2 out]
          n332 = property on="Play Button" class="Bool (strict)"("DisabledEnum"=w660) -> ()  [unwired: 2 in, 2 out]
        }
        n333 = while {
          shift-right: [w711] -> _
          shift-left: w646 -> [w710]
          shift-right: [w705] -> _
          shift-left: w645 -> [w709]
          shift-right: [w702] -> w632
          shift-left: w643 -> [w708]
          tunnel: [w707] -> w650
          tunnel: [w706] -> w649
          tunnel: w636 -> [w692]
          tunnel: w635 -> [w691]
          i -> [w699]
          stop <- w688 stop-if-true
          # "Attempt to slow down frame rate"
          n334 = call <vilib>:"IMAQdx Grab2.vi"("error in"=w708, "Image In"=w709, "Session In"=w710) -> ("error out"=w704:errorcluster, "Image Out"=w705:T1, "Session Out"=w711:T8)  [unwired: 5 in, 1 out]
          n335 = call <extravilib>:"Read.vi"("channel"=w691) -> ("element"=w690:bool)  [unwired: 1 in, 1 out]
          n336 = call <extravilib>:"Read.vi"("channel"=w692) -> ("element"=w689:bool)  [unwired: 1 in, 1 out]
          n337 = Quotient & Remainder(x=w699, y=4) -> (x-y*floor(x/y)=w697:i32)  [unwired: 1 out]
          n338 = Equal To 0?(x=w697) -> (x = 0?=w693:bool)
          n339 = Or(x=w693, y=TRUE) -> (x .or. y?=w696:bool)
          n340 = call "IMAQ Resample"("X Resolution"=960, "Y Resolution"=540, "error in (no error)"=w704, "Image Src"=w705) -> ("error out"=w703:errorcluster, "Image Dst Out"=w694:T1)  [unwired: 6 in]
          n341 = Or(x=w690, y=w689) -> (x .or. y?=w688:bool)
          n342 = case shown="True" w696 {
            tunnel: [_ w722] -> w707
            tunnel: [_ w717] -> w706
            tunnel: w688 -> [_ w713]
            tunnel: w703 -> [w712 w716]
            tunnel: [w712 w715] -> w702
            tunnel: w694 -> [_ w714]
            frame False {
            }
            frame True {
              n343 = Format Date/Time String(time format string (%c)="%H%M%S%3u") -> (date/time string=w719:string)  [unwired: 2 in]
              n344 = call "IMAQ ColorImageToArray"("Image"=w714, "error in (no error)"=w716) -> ("Image Pixels (U32)"=w723:u32[][], "error out"=w715:errorcluster)  [unwired: 2 in, 1 out]
              n345 = Concatenate Strings(w719, ".png" ("string")) -> (w718:string)
              n346 = call <extravilib>:"Write.vi"("last element? (F)"=w713, "element"=w723) -> ("channel"=w722:T14)  [unwired: 7 in, 2 out]
              n347 = call <extravilib>:"Write.vi"("last element? (F)"=w713, "element"=w718) -> ("channel"=w717:T15)  [unwired: 7 in, 2 out]
            }
          }
        }
        n348 = local write "Play Button"(w629) -> ()
        n349 = local write "Calibrate"(w629) -> ()
        n350 = local write "Close Program"(w629) -> ()
        n351 = local write "Save Button"(w629) -> ()
        n352 = local write "Pause Button"(w629) -> ()
        n353 = call "IMAQ Create"("Image Name"="Endoscope Consumer", "Image Type"=w647) -> ("New Image"=w648:T1)  [unwired: 3 in, 1 out]
        n354 = while {
          tunnel: w650 -> [w687]
          tunnel: w649 -> [w686]
          shift-right: [w679] -> _
          shift-left: w648 -> [w684]
          stop <- w677 stop-if-true
          # "Take filename from channel"
          # "Take image from channel"
          # "Save the image to file"
          # "Reads image from channel, converts it into an image, then writes that image to file."
          n355 = local read "WideField Path"() -> (w683:path)
          n356 = call <extravilib>:"Read.vi"("channel"=w686) -> ("element"=w682:string)  [unwired: 6 in, 4 out]
          n357 = call <extravilib>:"Read.vi"("channel"=w687) -> ("done?"=w677:bool, "element"=w685:u32[][])  [unwired: 6 in, 3 out]
          n358 = call "IMAQ ArrayToColorImage"("Image Pixels (U32)"=w685, "Image"=w684) -> ("Image Out"=w680:T1)  [unwired: 3 in, 1 out]
          n359 = Build Path(base path=w683, name or relative path=w682) -> (appended path=w678:path)
          n360 = call-poly "IMAQ Write File 2"("Image Quality"=u32 1000, "File Path"=w678, "Image"=w680) -> ("Image Out (duplicate)"=w679:T1)  [unwired: 7 in, 1 out]
        }
      }
      frame "Exit" {
        # "Log Program Finished"
        # "Tell the python program to close"
        n361 = Bundle By Name(cluster=T6 {"Source"="", "Destination"="", "CMD"="newfolders", "Time"="time"} ("Output JSON File"), "CMD"="stop") -> (w736:T6)
        n362 = local read "Command File Location"() -> (w733:path)
        n363 = Flatten To JSON(anything=w736, error in (no error)=w731) -> (JSON string=w735:string, 11:w734:errorcluster)  [unwired: 1 in]
        n364 = Write to Text File(file (use dialog)=w733, text=w735, error in=w734) -> (error out=w730:errorcluster)  [unwired: 1 in, 2 out]
        n365 = local read "Log File Out"() -> (w728:refnum<file>)
        n366 = call "Esophageal_Datalogger_EndButton.vi"("error in (no error)"=w730, "Log File In"=w728) -> ("error out"=w729:errorcluster)  [unwired: 8 in, 1 out]
      }
    }
    "Software States" <- w33
    "error out" <- w25
  }
  n367 = property on="Play Button" class="Bool (strict)"("DisabledEnum"=w3) -> ()  [unwired: 2 in, 2 out]
  n368 = property on="Calibrate" class="Bool (strict)"("DisabledEnum"=w3) -> ()  [unwired: 2 in, 2 out]
  n369 = property on="Save Button" class="Bool (strict)"("DisabledEnum"=w3) -> ()  [unwired: 2 in, 2 out]
  n370 = property on="Close Program" class="Bool (strict)"("DisabledEnum"=w3) -> ()  [unwired: 2 in, 2 out]
  n371 = property on="Auto Exposure" class="Bool (strict)"("DisabledEnum"=w3) -> ()  [unwired: 2 in, 2 out]
  n372 = property on="Auto Gain" class="Bool (strict)"("DisabledEnum"=w3) -> ()  [unwired: 2 in, 2 out]
  n373 = property on="Image Analysis Meter" class="Slide (strict)"("BG Color"=u32 0 ("Slider Colors:BG Color")) -> ()  [unwired: 2 in, 2 out]
  n374 = call <vilib>:"DAQmx Clear Task.vi"("task in"=w10, "error in"=w9) -> ("error out"=w1:errorcluster)  [unwired: 13 in]
  n375 = Close Python Session(session in=w2, error in=w1) -> ()  [unwired: 1 out]
